vi "Commercial2 Dryer Tool.vi"() -> ()   [LabVIEW 2023]
uses:
  Common/LabVIEW GEA2 Toolkit/GEA3/type defs/Data In.ctl
  Common/LabVIEW GEA2 Toolkit/GEA3/type defs/Source_Destination.ctl
  Common/LabVIEW GEA2 Toolkit/GEA3/type defs/ERD Write Data In.ctl
  Common/LabVIEW GEA2 Toolkit/GEA3/type defs/Data Type.ctl
  Common/LabVIEW GEA2 Toolkit/GEA3/type defs/ERD Read Data Out.ctl
  Common/LabVIEW GEA2 Toolkit/GEA3/type defs/ERD Read Data In.ctl
  Common/type defs/Programming.ctl
  Common/type defs/Flash_Results.ctl
  JL Dryer Tool Support/type defs/Cycle Control.ctl
  JL Dryer Tool Support/type defs/ERD_Always_Show_JL.ctl
  Common/GEA2 Script/typedefs/Script Info.ctl
  JL Dryer Tool Support/type defs/Relay_Control.ctl
  JL Dryer Tool Support/type defs/Drum_Light_Control.ctl
  <vilib>/Platform/fileVersionInfo.llb/FileVersionInformation.ctl
  Common/type defs/Choose_ERD_List.ctl
  Common/Diagnostics Decode/Type Defs/Diag_FaultTableStatus.ctl
  Common/Diagnostics Decode/Type Defs/Diag_FaultTableEntry.ctl
  Common/Diagnostics Decode/Type Defs/Diag_EntityManifestType.ctl
  Common/Diagnostics Decode/Type Defs/Diag_FaultSeqEntry.ctl
  Automation2/Product Specific/Clothes Care/Justice League/Product Testcode/Diagnostics/TypeDefs/Centauro Diagnostic V3 SnapShot.ctl
  JL Dryer Tool Support/type defs/JL_Diagnost V3 Cycle History.ctl
  Common/type defs/ERDList.ctl
  Common/type defs/ERD_Loop_States.ctl
  JL Dryer Tool Support/type defs/ERD_Commercial_Laundry.ctl
  JL Dryer Tool Support/type defs/ERD_RJ45.ctl
  Common/type defs/Version.ctl
  Common/type defs/BootloaderVersion.ctl
  Common/LabVIEW GEA2 Toolkit/GEA3/type defs/Data Out.ctl
  Common/type defs/ERD_Data_Loop_Control.ctl
  Common/type defs/Error_Command.ctl
  JL Dryer Tool Support/type defs/All_Bundled_Data_JL.ctl
  Common/type defs/CSV_File_String_Arrays.ctl
  Common/type defs/Fault Table Array.ctl
  Common/type defs/Fault_Table_Info.ctl
  JL Dryer Tool Support/type defs/Heat Control.ctl
  Common/GExplorer Support/typedefs/GExplorer_Data_Cluster.ctl
  JL Dryer Tool Support/type defs/DAQ_Control_Command.ctl
  Common/type defs/ERD_Loop_Control_Command.ctl
  Common/type defs/GEA2_Control_Command.ctl
  Common/LabVIEW GEA2 Toolkit/GEA3/advanced/GEA2 Message Received Event Handler.vi
  D:/Common/LabVIEW GEA2 Toolkit/source/GEA3 DLL Source/GeaCommunication.dll
  Common/LabVIEW GEA2 Toolkit/source/GEA3 DLL Source/GeaCommunication.dll
  Common/LabVIEW GEA2 Toolkit/GEA3/library/GEA2_Toolkit.lvlib
panel:
  out "Message":string
  in  "EndOfCycle":bool
  in  "Board Index":u8=1 max=10 step=1
  in  "Pause(mls)":u32=100
  out "Rate":u32=100
  out "State":T1=enum."Read ERDs"
  out "ERD_Always Show":T2={"Inlet Thermistor"=0, "Machine State"="IDLE", "Filtered Moisture"=0, "Cycle Selected"="", "HTR 1 / Inner / Top"=FALSE, "HTR 2 / Outer / Bot"=FALSE, "Door Switch"=FALSE, "Drum Light"=FALSE, "Cycle Engine State"="", "Centrifugal Switch"=FALSE, "Drum Motor"=FALSE, "Cycle Count"=0, "Ext. Tumble"=FALSE, "eDry"=FALSE, "Temp Level"="", "Dryness Level"="", "Time Level"="", "Delay Time (min)"=0, "Steam Refresh"=FALSE, "Damp Alert"=FALSE, "Sub-Cycle"="", "Outlet Thermistor"=0, "Target Moisture"=0, "Remaining Cycle Time"=0, "Raw Moisture"=0, "Cycle Name"="", "My Cycle"=FALSE, "Delay Dry"=FALSE, "Detangle"=FALSE, "Control Lock"=FALSE, "Steam Valve"=FALSE, "Door Latch"=FALSE, "Signal Volume"="", "Tune ID"="", "Restr Detect Status"="", "Vent Restriction"="", "Load Size by Contact"="", "Load Size by Temp"="", "EOC Reason"="", "Sensor Dry Status"="", "Dampness State"="", "Target Voltage Reached"=FALSE, "TrimInhibitR1"=FALSE, "TrimInhibitR2"=FALSE, "TrimBothCoilInhibit"=FALSE, "NormalHeatControl"=FALSE, "HeatControl Request"=FALSE, "Cool Down Status"="", "EcoDryInhibitRelay1"=FALSE, "EcoDryInhibitRelay2"=FALSE, "ReverseDrumInhibitRelay1"=FALSE, "ReverseDrumInhibitRelay2"=FALSE, "OverTempHeaterInhibitRequest"=FALSE, "FallbackHeatControlMethodStatus"=FALSE, "IHC TimeSeconds"=0, "ECT TimeSeconds "=0, "SC Total Drying Time(S')"=0, "TTR Target Voltage (S')"=0, "TCT Drying Time (S's)"=0, "Drum Motor State"=enum."Off", "Load Size by Ag"="", "MaxFIletered Voltage"=0, "Dry Load Detection"="", "Min Sensing Elapse Sec"=0, "Time Multi Sec X100"=0, "Time Adder  Sec"=0, "Temp Multi EcoDry"="", "Temp Multi ExtraLow"="", "Temp Multi Low "="", "Temp Multi Medium"="", "Temp Multi High"="", "SmoothMoisture"=0, "Eco Dry SEL Status"="", "Eco Dry SEL Result"="", "Eco Dry Cont Status"="", "Eco Dry Relay1 Timer"="", "Eco Dry Relay2 Timer "="", "Eco Dry Stage 2 Tans "=0, "WiFiCommissioningPSt"="IDLE", "Payment Method"=""}
  out "Temp ADC":T3
  in  "Read Parametric":bool=TRUE
  in  "Data ON":bool=TRUE
  in  "Stop":bool
  in  "Reset":bool
  in  "UI Launch":bool
  in  "Tab Control":T4(tab)=enum."ERD List"
  in  "Phase.Authorized":bool
  in  "Phase.Reserved":bool
  in  "Phase.Idle":bool
  in  "Residencial":bool
  out "Personality Set":u8=1
  in  "?":u8=1
  in  "Set Personality":bool
  out "CSV File Log Path":path=path "D:/QA/Commercial 2/Dryer_Xolo/ProbandoC2_24-11-21_15-05-37.csv"
  out "Commercial_Laundry":T5
  out "RJ45":T6
  out "Version":T7
  in  "Read ERD List":T8[](array[typedef])=[{"ERD Number"=49, "Data Type"=enum."string"}] {"ERD Number" format="%.0x"}
  in  "Read ERD":bool
  in  "Write ERD List":T9[](array[typedef])=[{"ERD Number"=49, "Data Type"=enum."string", "Data"="01"}] {"ERD Number" format="%.0x"}
  in  "Write ERD":bool
  out "Read ERD Data Out":T11[](array[typedef])=[{"ERD Number"=49, "Data"="00 00 00 16"}] {"ERD Number" format="%.0x"}
  out "Boot Loader Version":T12
  in  "GEA Inputs":T13={"Source"=229, "Destination"=192} {"Destination" format="%.0x"; "Source" format="%.0x"}
  out "Increment Price":T14={"DELICATE"=0.0, "LOW"=0.0, "MEDIUM"=0.5, "HIGH"=0.25} {"HIGH" min=0.0 max=9.75 step=0.25; "MEDIUM" min=0.0 max=9.75 step=0.25; "LOW" min=0.0 max=9.75 step=0.25; "DELICATE" min=0.0 max=9.75 step=0.25}
  out "Base Price":T14={"DELICATE"=0.0, "LOW"=0.0, "MEDIUM"=0.5, "HIGH"=0.25} {"HIGH" min=0.0 max=9.75 step=0.25; "MEDIUM" min=0.0 max=9.75 step=0.25; "LOW" min=0.0 max=9.75 step=0.25; "DELICATE" min=0.0 max=9.75 step=0.25}
  in  "See Price":bool
  in  "IncrementPrices":T14={"DELICATE"=0.0, "LOW"=0.25, "MEDIUM"=0.5, "HIGH"=0.25} {"HIGH" min=0.0 max=9.75 step=0.25; "MEDIUM" min=0.0 max=9.75 step=0.25; "LOW" min=0.0 max=9.75 step=0.25; "DELICATE" min=0.0 max=9.75 step=0.25}
  in  "SetIncrementPrices":bool
  in  "BasePrices":T14={"DELICATE"=0.0, "LOW"=0.0, "MEDIUM"=0.5, "HIGH"=0.25} {"HIGH" min=0.0 max=9.75 step=0.25; "MEDIUM" min=0.0 max=9.75 step=0.25; "LOW" min=0.0 max=9.75 step=0.25; "DELICATE" min=0.0 max=9.75 step=0.25}
  in  "Set Price":bool
  out "Increment Time":T15 {"HIGH" max=10 step=1; "MEDIUM" max=10 step=1; "LOW" max=10 step=1; "DELICATE" max=10 step=1}
  out "Base Time":T15 {"HIGH" max=10 step=1; "MEDIUM" max=10 step=1; "LOW" max=10 step=1; "DELICATE" max=10 step=1}
  in  "See Times":bool
  in  "Time Increment":T14={"DELICATE"=0.0, "LOW"=0.0, "MEDIUM"=1.0, "HIGH"=0.0} {"HIGH" min=0.0 max=90.0 step=1.0; "MEDIUM" min=0.0 max=90.0 step=1.0; "LOW" min=0.0 max=90.0 step=1.0; "DELICATE" min=0.0 max=90.0 step=1.0}
  in  "SetTimeIncrement":bool
  in  "Time Base":T16={"DELICATE"=0.0, "LOW"=10.0, "MEDIUM"=10, "HIGH"=10} {"HIGH" min=10 max=90 step=1; "MEDIUM" min=10 max=90 step=1; "LOW" min=10.0 max=90.0 step=1.0; "DELICATE" min=0.0 max=90.0 step=1.0}
  in  "Set Base Time":bool
  out "OK?":bool
  in  "Parametric":T17(ring)
  in  "Exit Botloader":bool
  in  "Enum":enum16{"All", "MC", "UI"}(ring)
  in  "Entry Botloader":bool
  out "FileVersionInfo":T18
  out "LabView/Version Number":string
  in  "Tool Version":bool=TRUE
  in  "Clear":bool
  in  "Programming":T19={"Program"=FALSE, "File Path"=path "", "Program Ind"=FALSE, "Reset Board"=FALSE, "Enter Bootloader"=FALSE, "Result"=9} {"Result" items=["ImageRejected", "BoardNotFound", "UnableToGetGeaConfiguration", "WriteToFlashNotAllowed", "ImageDownloadedSuccessfully", "ImagePresent", "WriteToFlashFailed", "EraseFailed", "CrcFailed", ""]}
  in  "Flash Latest":bool
  in  "Send Button":bool
  in  "GEA2 Send":T21={"Source"=228, "Destination"=192, "Command"=0, "Message"=""} {"Command" format="%02x"; "Destination" format="%02x"; "Source" format="%02x"}
  out "Converted Data Out":T22 {"CRC" format="%04x"; "Length" format="%02x"; "Command" format="%02x"; "Destination" format="%02x"; "Source" format="%02x"}
  in  "Write parametric":bool
  in  "Message to send":string="04 03"
  in  "Get Faults":bool
  in  "Clear Fault Table Buffer":bool
  in  "Clear Fault Seq Buffer":bool
  out "Fault Sequence Entries":T23[](array[typedef])
  out "Fault Seq Status":T24
  out "Fault Table Entries":T25[](array[typedef])
  out "Fault Table Status":T24
  out "Diagnostic Entity Manifest":T26
  out "Major Version":u8
  out "Minor Version":u8
  out "Fault Set?":bool
  in  "Filter by Count":bool=TRUE
  out "Centauro Fault Snapshot":T27
  in  "Drum Light":T28={"Drum Light ON"=FALSE, "Drum Light OFF"=FALSE, "On Time (s)"=5.0} {"On Time (s)" min=0.0 max=3600.0}
  in  "Relay Control":T29
  in  "LED Control":T30
  in  "Cycle Control":T31
  out "Sensor Dry Status":string
  out "Dampness State":string
  in  "Enable CC Mode":bool
  in  "Completed Cycles":u16
  in  "Requested Cycles":u16
  in  "TimeBetween Cycles":u32
  in  "Enabled":u8
  in  "ERD Spam GEA Inputs":T13={"Source"=229, "Destination"=192} {"Destination" format="%.0x"; "Source" format="%.0x"}
  in  "Get Cycle Data":bool
  in  "Filter by Status Count":bool=TRUE
  out "JL Cycle History":T32
  out "output cluster":T24
  in  "Script Log Path":path
  in  "Run Script":bool
  out "Script Pass/Fail?":bool
  out "Script Report Text":string
  in  "stop script":bool
  in  "Script Path":path
  out "Script Info":T33 {"Overall Script File Progress" scale=0.0..1.0; "Elapsed time (s)" format="%#.1f"; "Current Script Progress" scale=0.0..1.0}
  out "Script Error Out":errorcluster
  in  "Load ERD List":T34
  in  "ERD Default List":T35=[{"Boolean"=TRUE, "ERD Number"=8192, "ERD Nanme"="Erd_MachineStatus", "Data_Type"=enum."string"}, {"Boolean"=TRUE, "ERD Number"=65281, "ERD Nanme"="Erd_Personality", "Data_Type"=enum."string"}, {"Boolean"=TRUE, "ERD Number"=65423, "ERD Nanme"="Erd_EnterConsumerErrorMode", "Data_Type"=enum."string"}, {"Boolean"=TRUE, "ERD Number"=55, "ERD Nanme"="Erd_ServiceModeState", "Data_Type"=enum."string"}, {"Boolean"=TRUE, "ERD Number"=61811, "ERD Nanme"="EErd_WiFiCommissioningOption", "Data_Type"=enum."string"}, {"Boolean"=TRUE, "ERD Number"=61823, "ERD Nanme"="Erd_WiFiCommissioningPresenterState", "Data_Type"=enum."string"}, {"Boolean"=TRUE, "ERD Number"=55, "ERD Nanme"="Erd_ServiceModeState", "Data_Type"=enum."string"}, {"Boolean"=TRUE, "ERD Number"=61811, "ERD Nanme"="Erd_WiFiCommissioningOption", "Data_Type"=enum."string"}, {"Boolean"=TRUE, "ERD Number"=65522, "ERD Nanme"="Erd_Rj45LockedAtLeastOnce", "Data_Type"=enum."string"}, {"Boolean"=TRUE, "ERD Number"=8351, "ERD Nanme"="Erd_CommercialLaundryStatus", "Data_Type"=enum."string"}, {"Boolean"=TRUE, "ERD Number"=8350, "ERD Nanme"="Erd_CommercialLaundryStatusExternal", "Data_Type"=enum."string"}, {"Boolean"=TRUE, "ERD Number"=8398, "ERD Nanme"="Erd_RJ45WriteAccessActual", "Data_Type"=enum."string"}, {"Boolean"=TRUE, "ERD Number"=8397, "ERD Nanme"="Erd_RJ45WriteAccessRequest", "Data_Type"=enum."string"}, {"Boolean"=TRUE, "ERD Number"=61976, "ERD Nanme"="Erd_CommercialPaymentMethod", "Data_Type"=enum."string"}, {"Boolean"=TRUE, "ERD Number"=61977, "ERD Nanme"="Erd_CommercialCoinPaymentStatusRequest", "Data_Type"=enum."string"}] {"ERD Number" format="%x"}
  in  "ERD's List Ticket Testing":T35 {"ERD Number" format="%x"}
  in  "Wifi State":T36(ring)
  in  "Set Wifi State(ERD 6003)":bool
  in  "Turn on Wifi":bool
  in  "Turn off Wifi":bool
  out "Wifi Network State":string
  out "Wifi Password":string
  out "Wifi Network Name":string
  out "Mac Address":string
  in  "Get Wifi Data":bool
  out "Error Out":errorcluster
  # "Personality"
  # "Residencial"
  # "Simular pago con aplicación 209E phase"
  # "Ver. 1.3"
  # "Set Base Prices"
  # "BASE"
  # "INCREMENT"
  # "Set Increment Prices"
  # "Set Time Base"
  # "BASE"
  # "INCREMENT"
  # "Set Time Increments"
  # "This controls destination of ERD Spam.\nYou should never change source unless\nyou want to see the spam in the GEA log."
  # "Continuous cycle Config"
  # "Wifi State is Writing to ERD 6003 and communicating with the wifi board directly.  It will remain in the state you wrote it to until another command is recieved. \n\nOnly Write to invalid if you are testing the board in Invalid state."
  # "After turning on Wifi , wait about 30 seconds and press the Get Wifi Data button.  Network state should be 1, apmode.\n\nAll this is doing is Writing the ERD 0xF115 Service Request to request connect, or disconnect."
  # "Contact:\n\nTerrance Bradford\nTerrance.Bradford@geappliances.com"
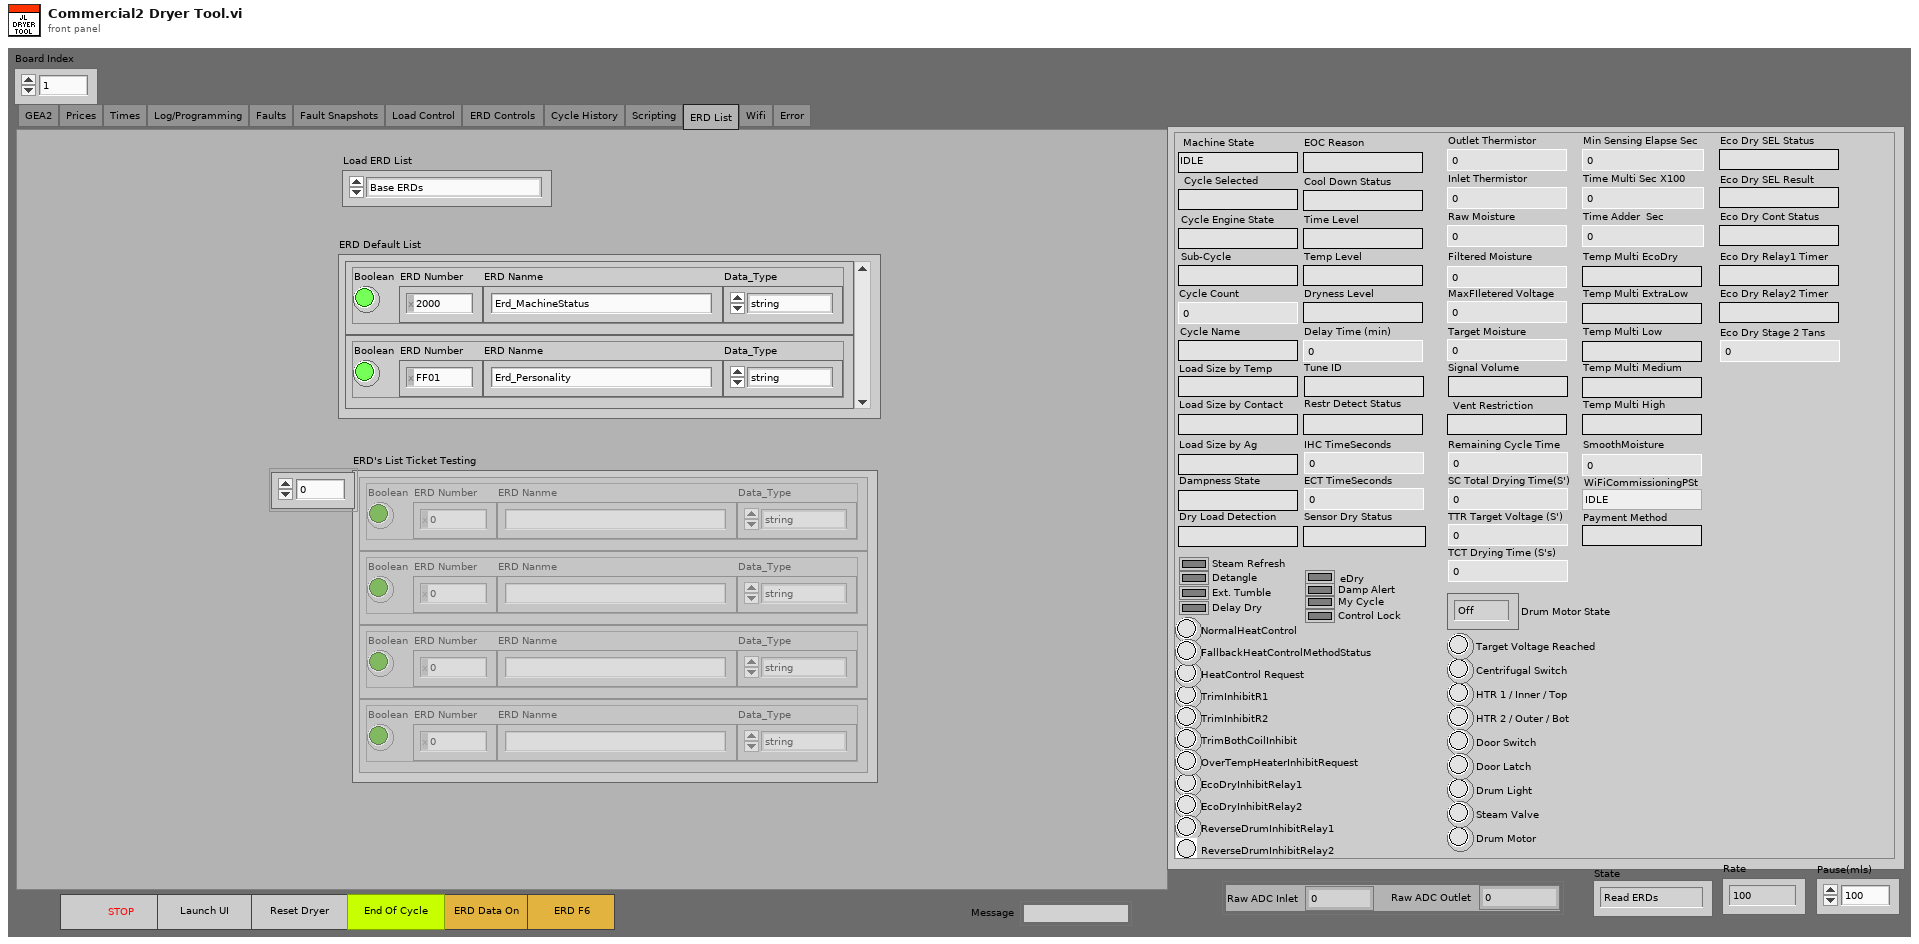
[diagram p1: front panel]
types:
  T1 = typedef "ERD_Loop_States.ctl" = enum16{"Init", "Build ERD Read List", "Read ERDs", "Get Version", "ERD´s User show", "Update UI", "Graph", "Read Faults", "Log Data", "Pause", "Shutdown"}
  T2 = typedef "ERD_Always_Show_JL.ctl" = cluster{"Inlet Thermistor":u16, "Machine State":string, "Filtered Moisture":u16, "Cycle Selected":string, "HTR 1 / Inner / Top":bool, "HTR 2 / Outer / Bot":bool, "Door Switch":bool, "Drum Light":bool, "Cycle Engine State":string, "Centrifugal Switch":bool, "Drum Motor":bool, "Cycle Count":u32, "Ext. Tumble":bool, "eDry":bool, "Temp Level":string, "Dryness Level":string, "Time Level":string, "Delay Time (min)":u16, "Steam Refresh":bool, "Damp Alert":bool, "Sub-Cycle":string, "Outlet Thermistor":u16, "Target Moisture":u16, "Remaining Cycle Time":u32, "Raw Moisture":u16, "Cycle Name":string, "My Cycle":bool, "Delay Dry":bool, "Detangle":bool, "Control Lock":bool, "Steam Valve":bool, "Door Latch":bool, "Signal Volume":string, "Tune ID":string, "Restr Detect Status":string, "Vent Restriction":string, "Load Size by Contact":string, "Load Size by Temp":string, "EOC Reason":string, "Sensor Dry Status":string, "Dampness State":string, "Target Voltage Reached":bool, "TrimInhibitR1":bool, "TrimInhibitR2":bool, "TrimBothCoilInhibit":bool, "NormalHeatControl":bool, "HeatControl Request":bool, "Cool Down Status":string, "EcoDryInhibitRelay1":bool, "EcoDryInhibitRelay2":bool, "ReverseDrumInhibitRelay1":bool, "ReverseDrumInhibitRelay2":bool, "OverTempHeaterInhibitRequest":bool, "FallbackHeatControlMethodStatus":bool, "IHC TimeSeconds":u32, "ECT TimeSeconds ":u32, "SC Total Drying Time(S')":u32, "TTR Target Voltage (S')":u32, "TCT Drying Time (S's)":u32, "Drum Motor State":enum16{"Off", "Cw", "Ccw", "Max"}, "Load Size by Ag":string, "MaxFIletered Voltage":u16, "Dry Load Detection":string, "Min Sensing Elapse Sec":u32, "Time Multi Sec X100":u32, "Time Adder  Sec":u32, "Temp Multi EcoDry":string, "Temp Multi ExtraLow":string, "Temp Multi Low ":string, "Temp Multi Medium":string, "Temp Multi High":string, "SmoothMoisture":u16, "Eco Dry SEL Status":string, "Eco Dry SEL Result":string, "Eco Dry Cont Status":string, "Eco Dry Relay1 Timer":string, "Eco Dry Relay2 Timer ":string, "Eco Dry Stage 2 Tans ":u32, "WiFiCommissioningPSt":string, "Payment Method":string}
  T3 = cluster{"Raw ADC Outlet":u16, "Raw ADC Inlet":u16}
  T4 = enum32{"GEA2", "Prices", "Times", "Log/Programming", "Faults", "Fault Snapshots", "Load Control", "ERD Controls ", "Cycle History", "Scripting", "ERD List", "Wifi", "Error"}
  T5 = typedef "ERD_Commercial_Laundry.ctl" = cluster{"Session":string, "Phase":string, "Appliance Type":string, "Cycle Selected":string, "Platform Type":string, "Retry Signal":string, "Session Ext":string, "Phase Ext":string, "Appliance Type Ext":string, "Cycle Selected Ext":string, "Platform Type Ext":string, "Retry Signal Ext":string}
  T6 = typedef "ERD_RJ45.ctl" = cluster{"Write Access Actual":string, "Write Access Request":string, "LockedAtLeastOnce":string}
  T7 = typedef "Version.ctl" = cluster{"Build Number":string, "Build Hash ":string, "Application Version":string, "Parametric Version":string, "UI App Version":string}
  T8 = typedef "ERD Read Data In.ctl" = cluster{"ERD Number":u16, "Data Type":enum16{"string", "boolean", "uint8_t", "uint16_t", "uint32_t", "uint64_t", "int8_t", "int16_t", "int32_t", "int64_t"}}
  T9 = typedef "ERD Write Data In.ctl" = cluster{"ERD Number":u16, "Data Type":T10, "Data":string}
  T10 = typedef "Data Type.ctl" = enum16{"string", "boolean", "uint8_t", "uint16_t", "uint32_t", "uint64_t", "int8_t", "int16_t", "int32_t", "int64_t"}
  T11 = typedef "ERD Read Data Out.ctl" = cluster{"ERD Number":u16, "Data":string}
  T12 = typedef "BootloaderVersion.ctl" = cluster{"UI BL Version":string, "MC BL Version":string}
  T13 = typedef "Source_Destination.ctl" = cluster{"Source":u8, "Destination":u8}
  T14 = cluster{"DELICATE":dbl, "LOW":dbl, "MEDIUM":dbl, "HIGH":dbl}
  T15 = cluster{"DELICATE":u32, "LOW":u32, "MEDIUM":u32, "HIGH":u32}
  T16 = cluster{"DELICATE":dbl, "LOW":dbl, "MEDIUM":u8, "HIGH":u8}
  T17 = enum16{"Board SKU", "Board Serial Number", "Unit SKU", "Unit Serial Number"}
  T18 = typedef "FileVersionInformation.ctl" = cluster{"FileVersion":string, "ProductName":string, "InternalName":string, "CompanyName":string, "LegalCopyright":string, "FileDescription":string}
  T19 = typedef "Programming.ctl" = cluster{"Program":bool, "File Path":path, "Program Ind":bool, "Reset Board":bool, "Enter Bootloader":bool, "Result":T20}
  T20 = typedef "Flash_Results.ctl" = i32
  T21 = typedef "Data In.ctl" = cluster{"Source":u8, "Destination":u8, "Command":u8, "Message":string}
  T22 = typedef "GEA2_Toolkit.lvlib/Data Out.ctl" = cluster{"Source":u8, "Destination":u8, "Command":u8, "Length":u8, "CRC":u16, "Message":string}
  T23 = typedef "Diag_FaultSeqEntry.ctl" = cluster{"Cycle #":u32, "Time":u32, "F Code":string, "F Active":bool}
  T24 = typedef "Diag_FaultTableStatus.ctl" = cluster{"Cur Index":u16, "Count":u16, "Ov Cnt":u16}
  T25 = typedef "Diag_FaultTableEntry.ctl" = cluster{"Cycle #":u32, "Time":u32, "F Code":string, "F Count":u16, "F Active":bool}
  T26 = typedef "Diag_EntityManifestType.ctl" = cluster{"ID":u8, "Data Ver Maj":u8, "Data Ver Min":u8, "Fault Table?":bool, "Fault Table Snap?":bool, "Fault Seq?":bool, "Fault Seq Snap?":bool, "Cycle History Seq?":bool, "Fault Table Entry Count":u16, "Fault Seq Entry Count":u16, "Cycle History Entry Count":u16, "Cycle Count":u32, "Entity Run Time (Min)":u32}
  T27 = typedef "Centauro Diagnostic V3 SnapShot.ctl" = string[][]
  T28 = typedef "Drum_Light_Control.ctl" = cluster{"Drum Light ON":bool, "Drum Light OFF":bool, "On Time (s)":dbl}
  T29 = typedef "Relay_Control.ctl" = cluster{"Drum Motor":bool, "HTR 2 / Outer / Bot":bool, "Steam Valve":bool, "Relays ON":bool, "Relays OFF":bool, "HTR 1 / Inner / Top":bool, "Pump":bool}
  T30 = cluster{"ALL LEDs ON":bool, "ALL LEDs OFF":bool, "Reset LEDs":bool}
  T31 = typedef "Cycle Control.ctl" = cluster{"Start Cycle":bool, "Cycle Selection":u8, "Stop Cycle":bool, "Pause Cycle":bool, "Resume Cycle":bool, "Select Cycle":bool}
  T32 = typedef "JL_Diagnost V3 Cycle History.ctl" = string[][]
  T33 = typedef "Script Info.ctl" = cluster{"Overall Script File Progress":dbl, "Current Script Progress":dbl, "Script":string, "Test":string, "Elapsed time (s)":dbl, "Done?":bool}
  T34 = typedef "Choose_ERD_List.ctl" = enum16{"Base ERDs", "QA ERDs", "MABE ERD List", "EcoDry Evaluation ERD List", "ClothDampnessCheck ERD List"}
  T35 = typedef "ERDList.ctl" = cluster{"Boolean":bool, "ERD Number":u16, "ERD Nanme":string, "Data_Type":enum16{"string", "boolean", "uint8_t", "uint16_t", "uint32_t", "uint64_t", "int8_t", "int16_t", "int32_t", "int64_t"}}[]
  T36 = enum16{"0 - OFF", "1 - App Mode", "2 - Connecting", "3 - Connected", "4 - Connected Off", "5 - Scanning", "6 - Reconnecting", "255 - Invalid"}
  T37 = typedef "All_Bundled_Data_JL.ctl" = cluster{"Version":T7, "ERD_Always Show":T2, "Personality Set":u8, "CSV File String Arrays":T38, "Fault Table Array ":T39, "Heat Control":T41, "Temp ADC":cluster{"Raw ADC Outlet":u16, "Raw ADC Inlet":u16}, "Commercial_Laundry":T5, "Boot Loader Version":T12, "RJ45":T6}
  T38 = typedef "CSV_File_String_Arrays.ctl" = cluster{"ERD Number Array":string[], "ERD Name Array":string[], "ERD Converted String Data":string[]}
  T39 = typedef "Fault Table Array.ctl" = T40[]
  T40 = typedef "Fault_Table_Info.ctl" = cluster{"Cycle Count":u32, " Runtime (min) ":u32, "Fault Status":string, "Fault ID":string, "Fault Count":u16}
  T41 = typedef "Heat Control.ctl" = cluster{"Htr1 InletLowLim":string, "Htr1 InletUpLim":string, "Htr1 OutletLowLim":string, "Htr1 OutletUpLim":string, "Htr1 FallBackON(s)":string, "Htr1 FallBackOFF(s)":string, "Htr1":bool, "Htr2 InletLowLim":string, "Htr2 InletUpLim":string, "Htr2 OutletLowLim":string, "Htr2 OutletUpLim":string, "Htr2 FallBackON(s)":string, "Htr2 FallBackOFF(s)":string, "Htr2":bool}
  T42 = typedef "ERD_Data_Loop_Control.ctl" = cluster{"Data":variant, "State":T1}
  T43 = typedef "Error_Command.ctl" = enum16{"Initialize", "Handle Errors", "Report Errors"}
  T44 = enum8{"Enabled", "Disabled", "Disabled and Grayed Out"}
  T45 = enum16{"UI Application APL", "UI Parametric APL", "MC APL"}
  T46 = typedef "GEA2_Control_Command.ctl" = enum16{"Initialize", "Shutdown"}
  T47 = typedef "ERD_Loop_Control_Command.ctl" = enum16{"Initialize", "Shutdown"}
  T48 = typedef "DAQ_Control_Command.ctl" = enum16{"Initialize", "Shutdown", "Exit"}
  T49 = typedef "GExplorer_Data_Cluster.ctl" = cluster{"Data":variant, "State":enum16{"Add to Log", "Clear", "Shutdown"}}
  T50 = typedef "F6_ERD_Control.ctl" = cluster{"EcoDryEnabledFlag":string, "KeyCycleId":u8, "CycleType":string, "Time LVL option 5":u32, "Time LVL option 4":u32, "Time LVL option _3":u32, "Time LVL option _2":u32, "Time LVL option _1":u32, "Time LVL option _0":u32, "CoolDownTimeInSeconds":u32, "TimeAdjustTimeCycleMinimumTimeInSeconds":u32, "TimeAdjustTimeCycleMaximumTimeInSeconds":u32, "TimeAdjustTimeCycleStandardAdjustTimeInSeconds":u32, "TimeAdjustTimeCycleSlewAdjustTimeInSeconds":u32, "ExtendedTumbleTimeInSeconds":u32, "SanitizeMaxDryTimeInSeconds":u32, "TemperatureDefault Level":u8, "Temperature ecoDryDefualtLevel":u8, "DrynessDefault Level":u8, "DrynessDefault ecoDryDefualtLevel":u8, "TimeAdjust defaultLevel":u8, "TimeAdjust ecoDryDefualtLevel":u8, "TimeLevelDefault Level":u8, "TimeLevelDefault Eco Dry":u8, "EStarSensorDry Default Level":u8, "EStarSensorDry ecoDryDefaultLevel":u8, "EcoDryDefault Level":u8, "EcoDryDefault EcoDryDefaultLevel ":u8, "ExtendedTumble Default Level":u8, "ExtendedTumble  EcoDryDefaultLevel":u8, "Sanitize Default Level":u8, "Sanitize ecoDryDefualtLevel":u8, "MyCycleDefault Level":u8, "MyCycleDefault ecoDryDefualtLevel":u8, "StartPause Default Level":u8, "StartPause ecoDryDefualtLevel":u8, "Power Default Level":u8, "Power ecoDryDefualtLevel":u8, "KeyVolume Default Level":u8, "KeyVolume ecoDryDefualtLevel":u8, "AlertVolume Default Level":u8, "AlertVolume ecoDryDefualtLevel":u8, "ControlLock Default Level":u8, "ControlLock EecoDryDefualtLevel":u8, "HeatControlRelay1EcoDryParametricDataEntry\nHeatControlTemperatureLimit_InletLower":u16, "HeatControlRelay1EcoDryParametricDataEntry\nHeatControlTemperatureLimit_InletUpper":u16, "HeatControlRelay1EcoDryParametricDataEntry\nHeatControlTemperatureLimit_OutletLower":u16, "HeatControlRelay1EcoDryParametricDataEntry\nHeatControlTemperatureLimit_OutletUpper":u16, "HeatControlRelay1EcoDryParametricDataEntry\nonTimeInSeconds":u8, "HeatControlRelay1EcoDryParametricDataEntry\noffTimeInSeconds":u8, "HeatControlRelay1EcoDryParametric\nDataEntryChange ":bool, "HeatControlRelay2 EcoDryParametricDataEntry\nHeatControlTemperatureLimit_InletLower":u16, "HeatControlRelay2 EcoDryParametricDataEntry\nHeatControlTemperatureLimit_InletUpper ":u16, "HeatControlRelay2EcoDryParametricDataEntry\nHeatControlTemperatureLimit_OutletLower ":u16, "HeatControlRelay2EcoDryParametricDataEntry\nHeatControlTemperatureLimit_OutletUpper":u16, "HeatControlRelay2EcoDryParametricDataEntry\nonTimeInSeconds ":u8, "HeatControlRelay2EcoDryParametricDataEntry\noffTimeInSeconds ":u8, "HeatControlRelay2EcoDry\nParametricDataEntryChange":bool, "DampAlert Default Level":u8, "DampAlert ecoDryDefaultLevel":u8, "Detangle Default Level ":u8, "Detangle ecoDryDefaultLevel":u8, "DelayStart Default Level":u8, "DelayStart ecoDryDefaultLevel":u8, "CycleAllowsInventoryChangeChange":bool, "TemperatureAllowable":u8, "DrynessAllowable":u8, "TimeLevelAllowable":u8, "EcoDryAllowable":u8, "ExtendedTumbleAllowable":u8, "DampAlertAllowable":u8, "DetangleAllowable":u8, "DelayStartAllowable":u8, "SanitizeAllowable":u8, "MyCycleAllowable":u8, "TimeAdjustAllowable":u8, "Power Allowable":u8, "KeyVolumeAllowable":u8, "AlertVolumeAllowable":u8, "ControlLockAllowable":u8, "EStarSensorDryAllowable":string, "StartPauseAllowable":u8, "EcoDryStage1Heater2\nActiveSeconds":u32, "EcoDryStage2PeriodSeconds":u32, "EcoDryStage2Heater1\nActiveSeconds":u32, "EcoDryStage2Heater2\nActiveSeconds":u32, "EcoDryStage1Heater1\nActiveSeconds":u32, "EcoDryStage1PeriodSeconds":u32, "EcoDryStage2DurationSeconds":u32, "CoolDownAdaptiveTargetTemperature":u16}
  T51 = enum32{"invalid app kind", "Development System", "Run Time System", "Student Edition", "Embedded LabVIEW", "Evaluation", "Custom"}
  T52 = cluster{"ERD Data Out[0]":cluster{"ERD Number":u16, "Data":string}, "ERD Data Out[1]":cluster{"ERD Number":u16, "Data":string}, "ERD Data Out[2]":cluster{"ERD Number":u16, "Data":string}, "ERD Data Out[3]":cluster{"ERD Number":u16, "Data":string}, "ERD Data Out[4]":cluster{"ERD Number":u16, "Data":string}, "ERD Data Out[5]":cluster{"ERD Number":u16, "Data":string}, "ERD Data Out[6]":cluster{"ERD Number":u16, "Data":string}, "ERD Data Out[7]":cluster{"ERD Number":u16, "Data":string}, "ERD Data Out[8]":cluster{"ERD Number":u16, "Data":string}}
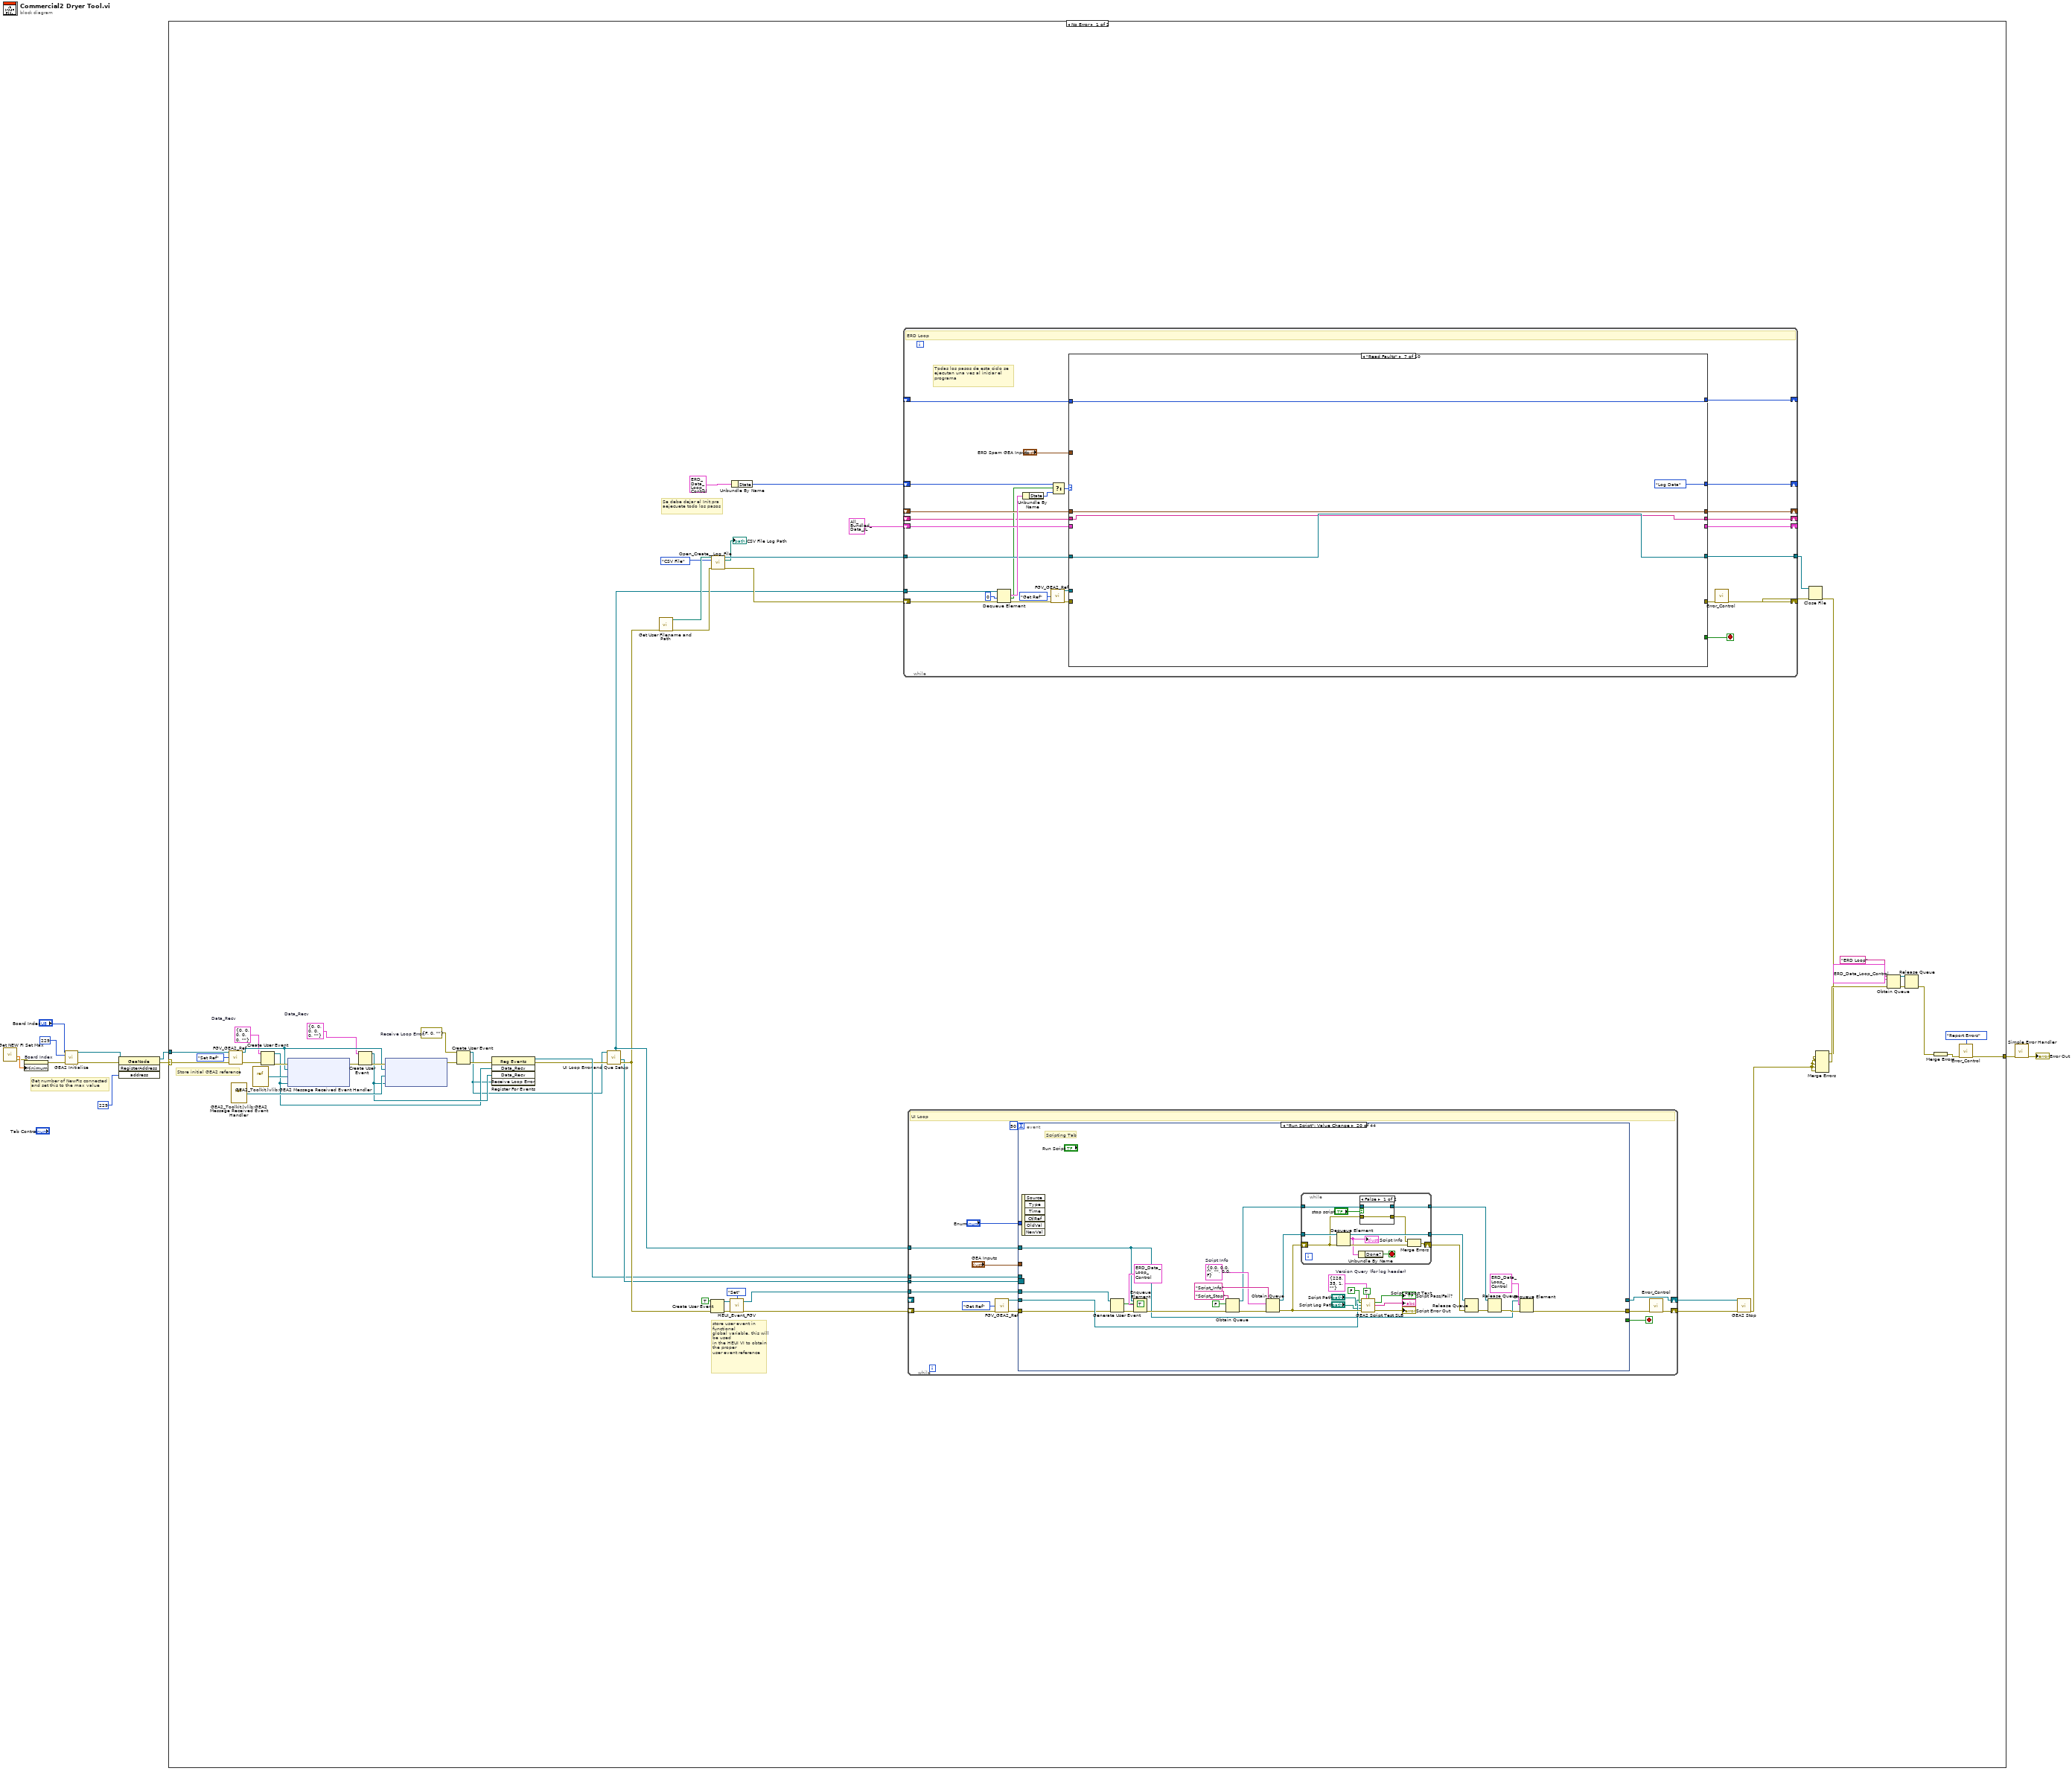
[diagram p0: block diagram]
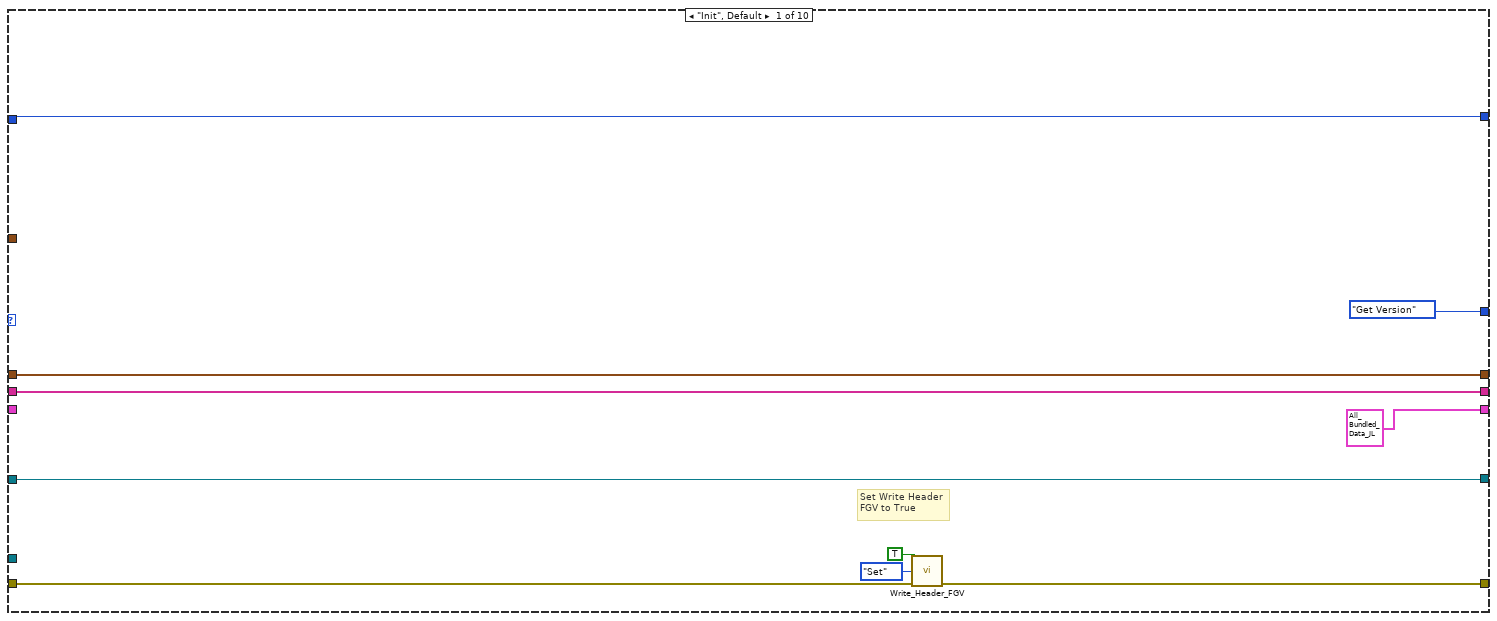
[diagram p2: hidden frame]
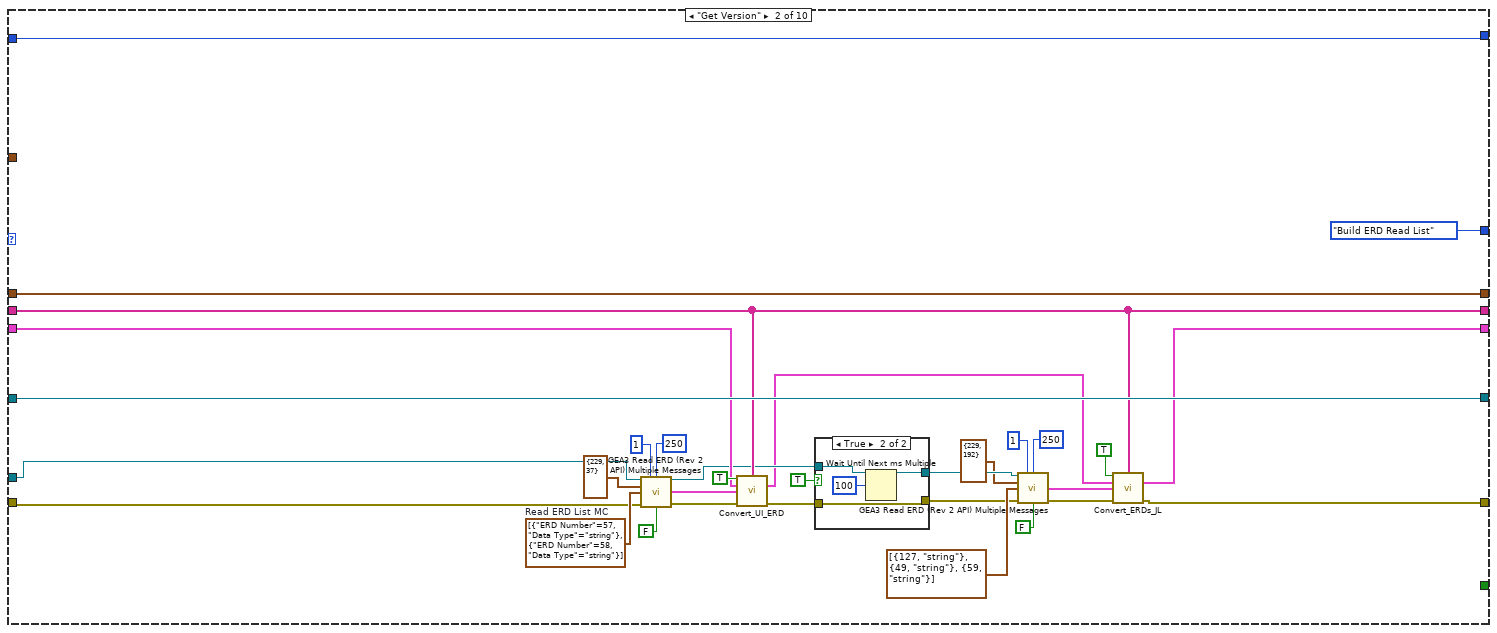
[diagram p3: hidden frame]
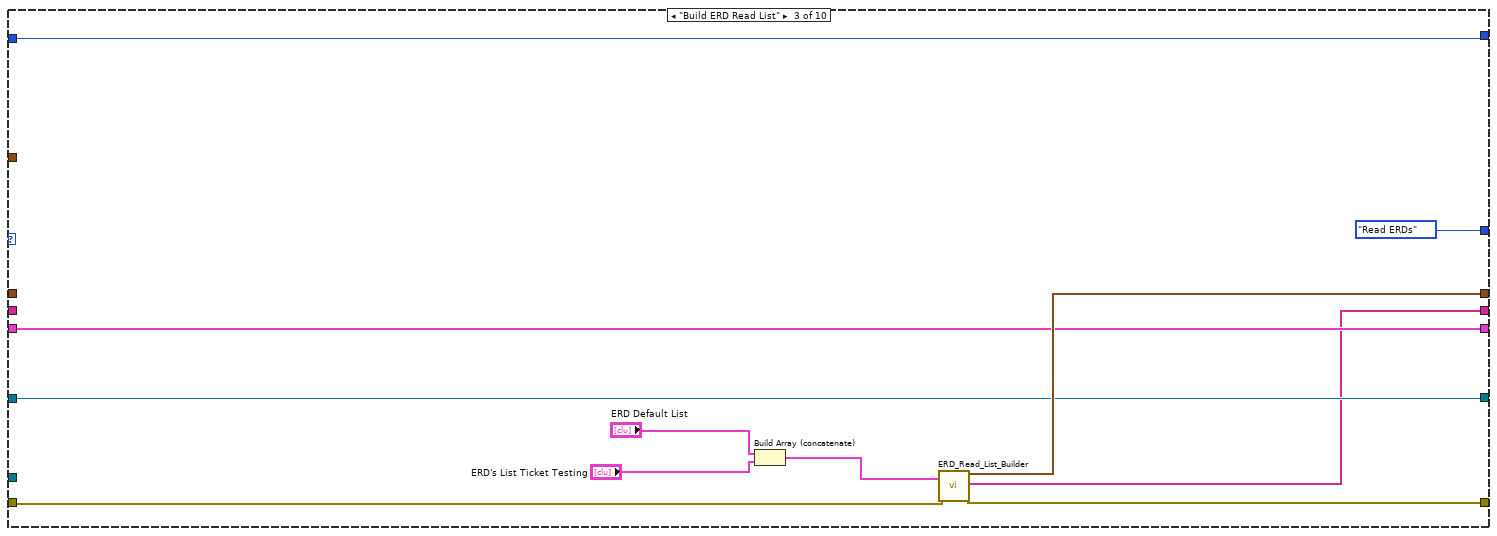
[diagram p5: hidden frame]
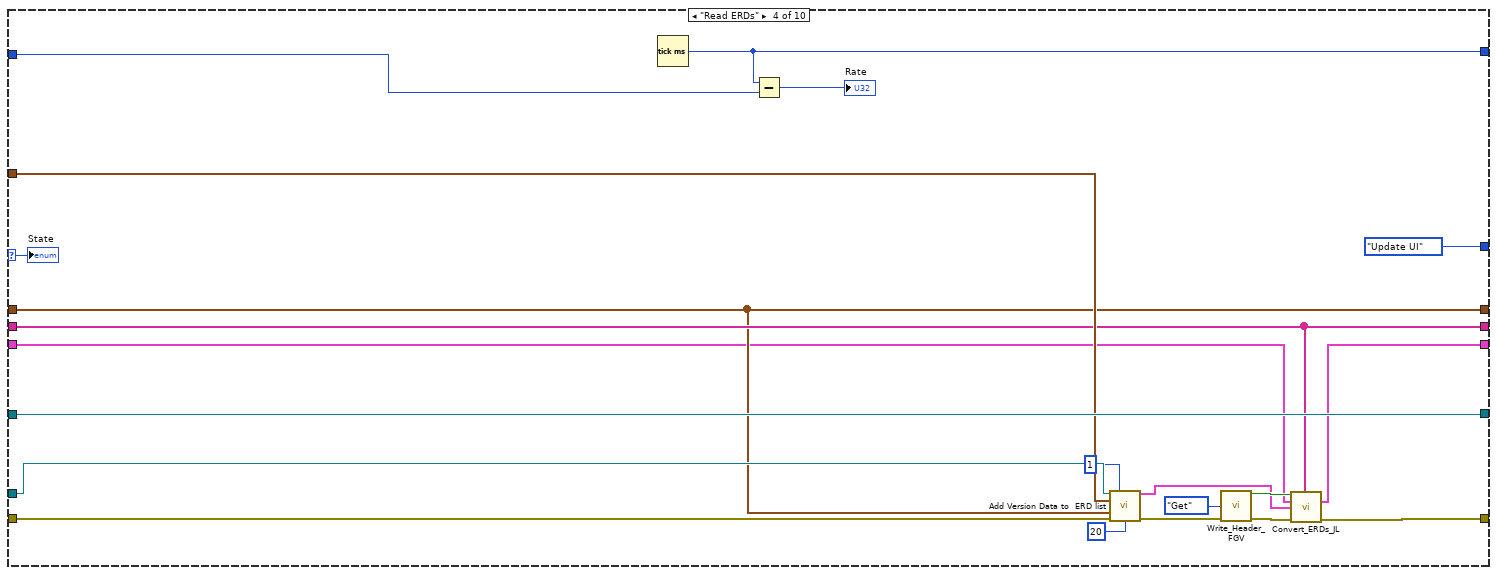
[diagram p6: hidden frame]
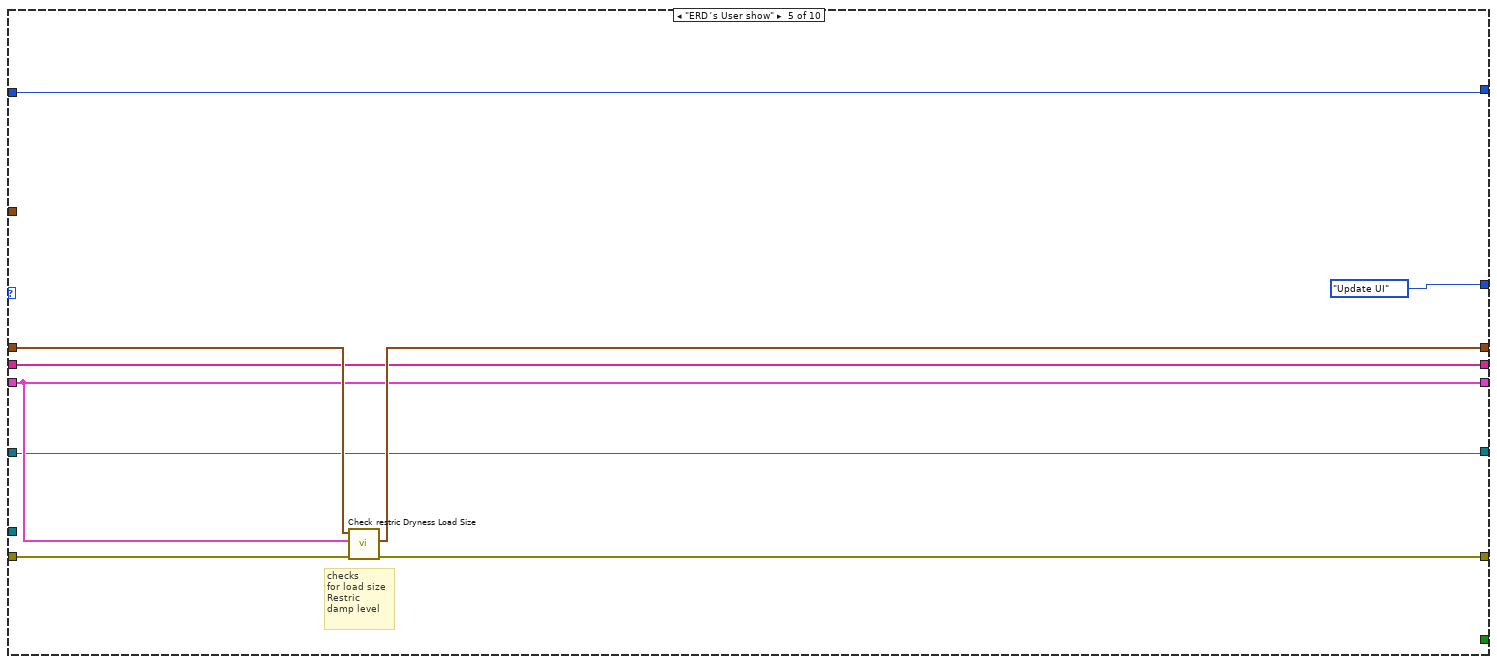
[diagram p7: hidden frame]
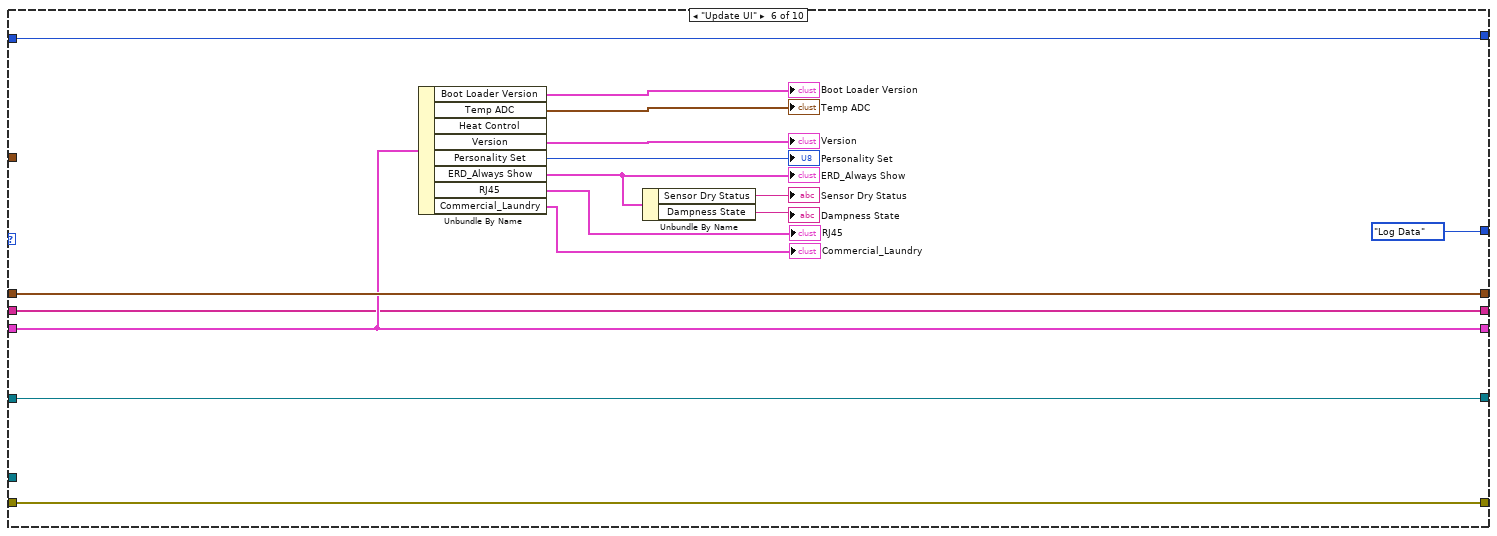
[diagram p8: hidden frame]
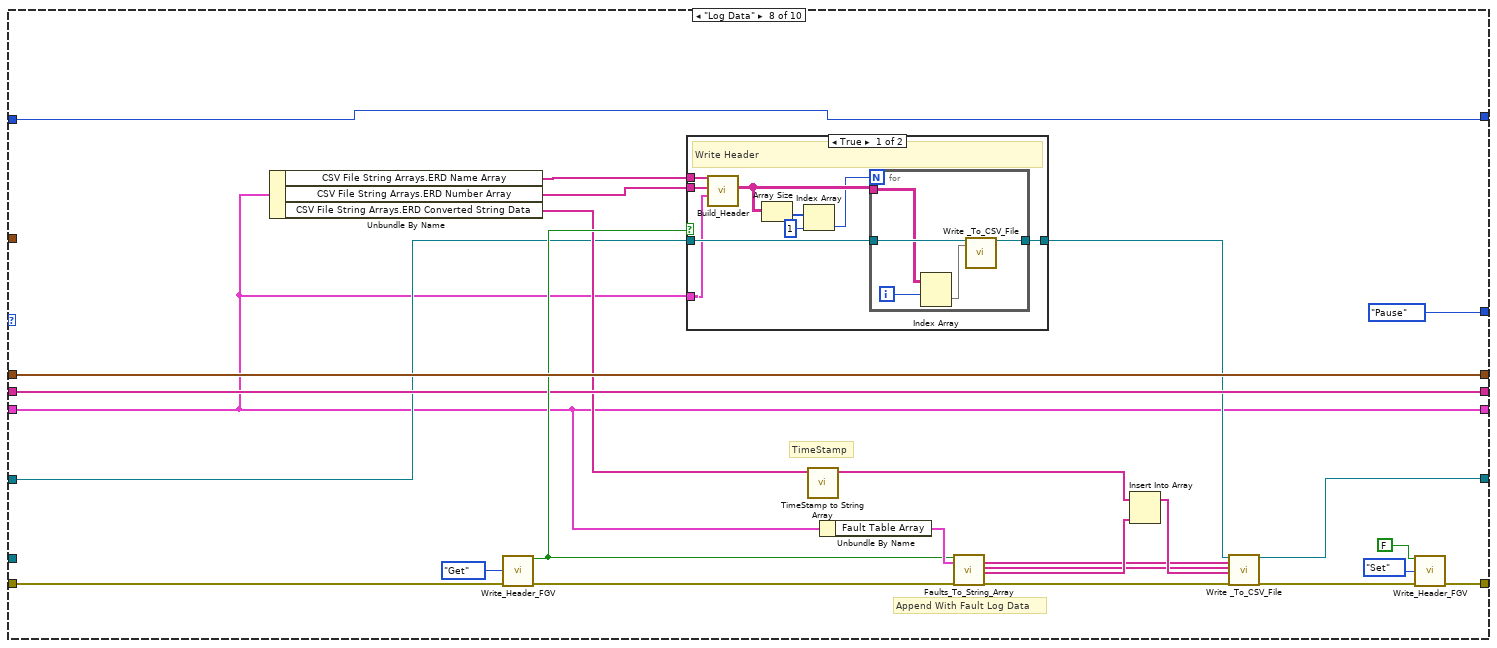
[diagram p9: hidden frame]
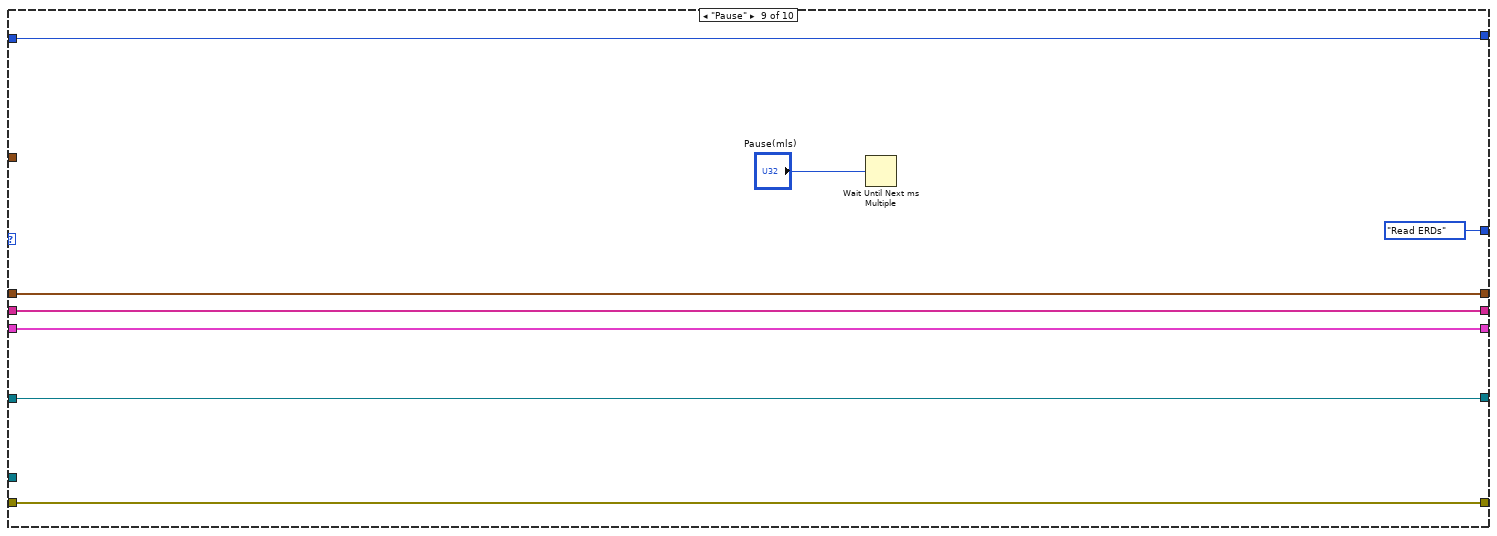
[diagram p11: hidden frame]
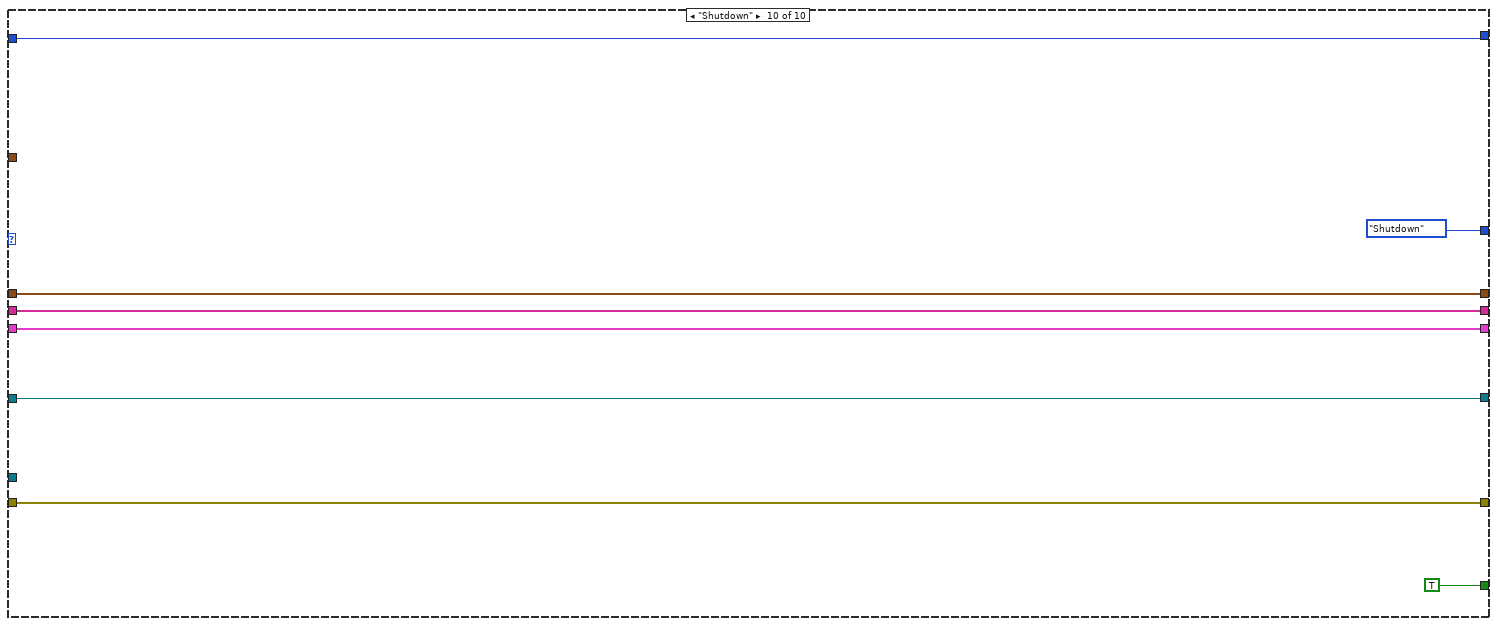
[diagram p12: hidden frame]
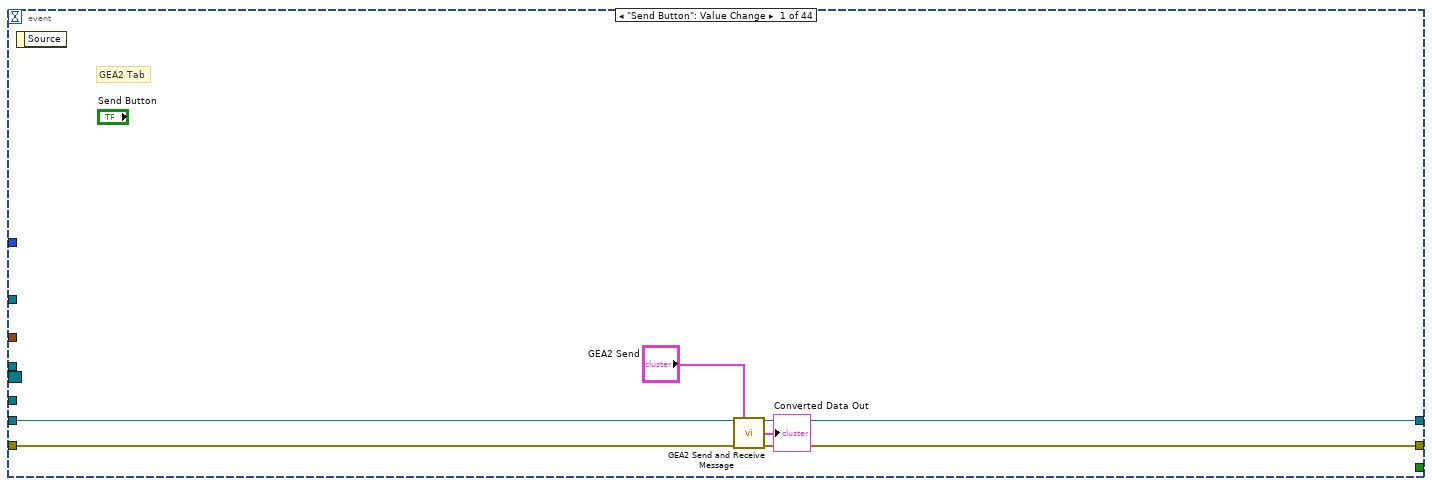
[diagram p13: hidden frame]
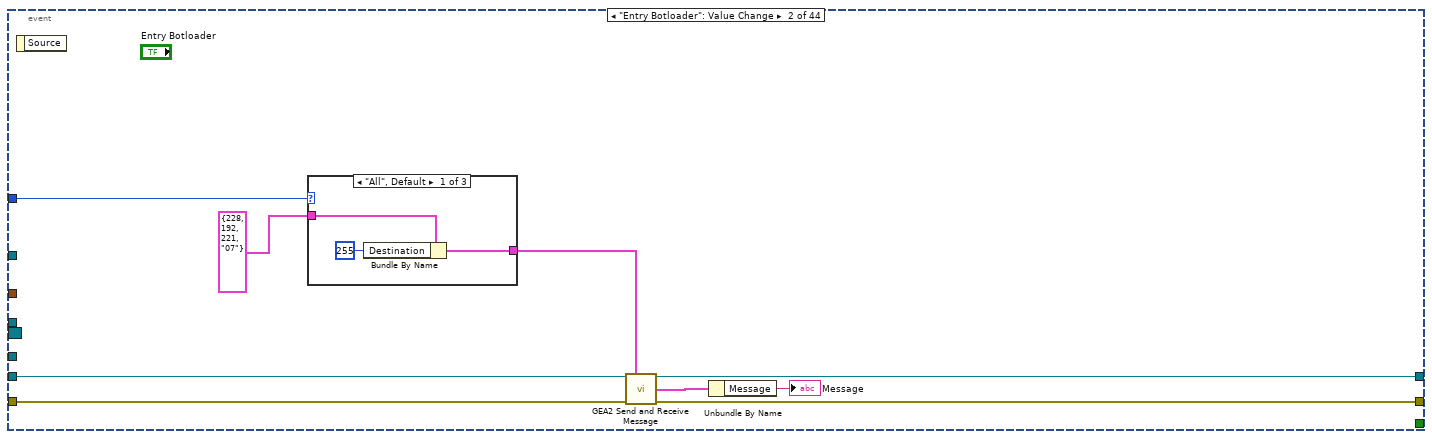
[diagram p14: hidden frame]
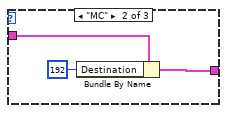
[diagram p15: hidden frame]
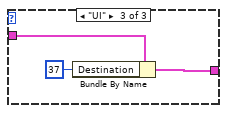
[diagram p16: hidden frame]
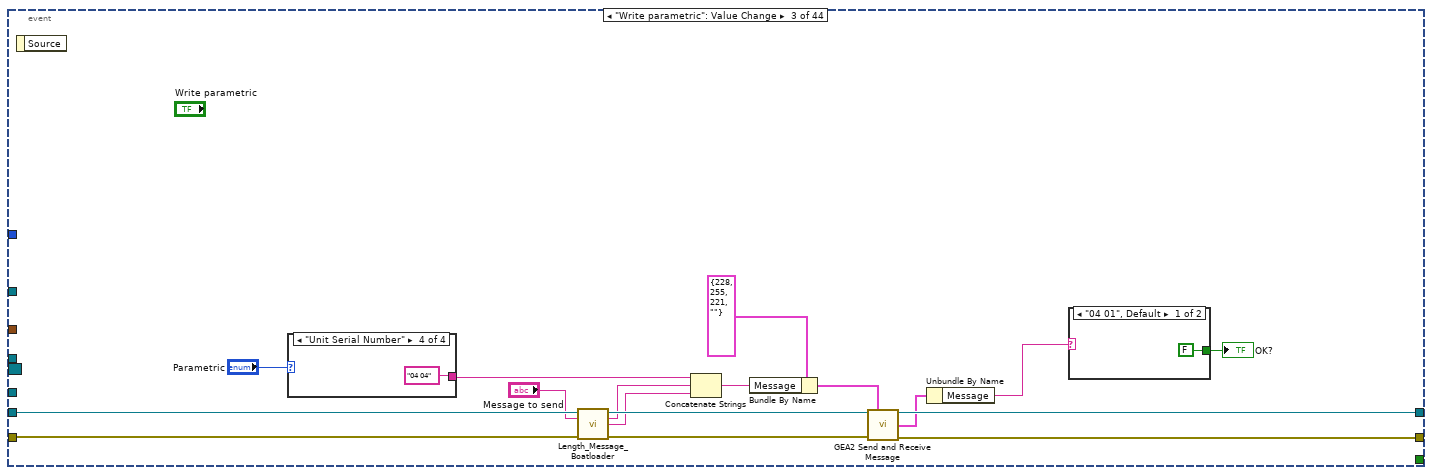
[diagram p17: hidden frame]
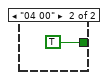
[diagram p18: hidden frame]
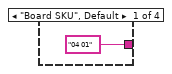
[diagram p19: hidden frame]
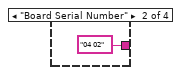
[diagram p20: hidden frame]
diagram:
  # "Get number of NewFIs connected\nand set this to the max value"
  n1 = call "Get NEW FI Set Max.vi"() -> ("Error Out"=w8:errorcluster, "Get Max_Out"=w9:dbl)  [unwired: 10 in]
  n2 = property on="Board Index" class="DigNum (strict)"(error in=w8, "Minimum"=w9) -> (error out=w7:errorcluster)  [unwired: 1 in, 1 out]
  n3 = call "GEA2 Initialize.vi"("Board Index"="Board Index", "Source Address"=u8 229, "error in"=w7) -> ("GEA2 Reference Out"=w5:refnum<k24>, "error out"=w2:errorcluster)  [unwired: 10 in, 1 out]
  n4 = invoke class="GeaNode" method="RegisterAddress"(reference=w5, error in=w2, "address"=u8 229 ("Source Address")) -> (reference out=w3:refnum<k24>, error out=w4:errorcluster)  [unwired: 1 in, 2 out]
  n5 = case shown="No Error" w4 {
    selector: w4 -> [w54 w1235]
    tunnel: [w55 w1235] -> w12
    tunnel: w3 -> [w33 _]
    frame No Error {
      w15 = T22 {"Source"=0, "Destination"=0, "Command"=0, "Length"=0, "CRC"=0, "Message"=""}  # Data_Recv
      w17 = T22 {"Source"=0, "Destination"=0, "Command"=0, "Length"=0, "CRC"=0, "Message"=""}  # Data_Recv
      w25 = errorcluster {"status"=FALSE, "code"=0, "source"=""}  # Receive Loop Error
      # "Se debe dejar el Init pra aejecuete todo los pasos"
      # "store user event in functional\nglobal variable, this will be used\nin the HEUI VI to obtain the proper\nuser event reference"
      # "Store initial GEA2 reference"
      n6 = call "FGV_GEA2_Ref.vi"("GEA2 Reference In"=w33, "Action"=enum16{"Set Ref", "Get Ref"}."Set Ref", "Error In"=w54) -> ("GEA2 Reference Out"=w28:refnum<k24>, "Error Out"=w16:errorcluster)  [unwired: 11 in]
      n7 = vi-ref "GEA2_Toolkit.lvlib:GEA2 Message Received Event Handler.vi"() -> (w26:refnum<vi>)
      n8 = vi-ref "GEA2_Toolkit.lvlib:GEA2 Message Received Event Handler.vi"() -> (w27:refnum<vi>)
      n9 = Create User Event(user event datatype=w17, error in=w16) -> (user event=w21:refnum<user-event>, error out=w30:errorcluster)
      n10 = node(w30, w28, w27, w21) -> (w31:errorcluster)  [unwired: 1 in, 1 out]
      n11 = Create User Event(user event datatype=w15, error in=w31) -> (user event=w22:refnum<user-event>, error out=w29:errorcluster)
      n12 = node(w29, w28, w26, w22) -> (w24:errorcluster)  [unwired: 1 in, 1 out]
      n13 = Create User Event(user event datatype=w25, error in=w24) -> (user event=w18:refnum<user-event>, error out=w23:errorcluster)
      n14 = register-events(error in=w23, w21, w22, w18) -> (reference out=w20:refnum<event-registration>, error out=w19:errorcluster)  [unwired: 1 in]
      n15 = call "UI Loop Error and Que Setup.vi"("error in (no error)"=w19, "Receive Loop"=w18) -> ("error out"=w34:errorcluster, "UI Loop Event Registration"=w32:refnum<event-registration>, "ERD Queue Loop"=w35:refnum<queue>)  [unwired: 6 in, 1 out]
      n16 = call "Get User Filename and Path.vi"("error in (no error)"=w34) -> ("error out"=w36:errorcluster, "CSV File Path"=w38:path)  [unwired: 8 in, 1 out]
      n17 = Create User Event(user event datatype=TRUE ("Bool"), error in=w34) -> (user event=w49:refnum<user-event>, error out=w50:errorcluster)
      n18 = call "Open_Create__Log_File.vi"("File Path Control"=w38, "Enum"=enum16{"CSV File", "Text File"}."CSV File", "Error In"=w36) -> ("refnum out"=w43:refnum<file>, "File Path"=→"CSV File Log Path":path, "Error Out"=w52:errorcluster)  [unwired: 10 in]
      n19 = call "HEUI_Event_FGV.vi"("Event In"=w49, "Action"=enum16{"Get", "Set"}."Set", "Error In"=w50) -> ("Event Out"=w46:refnum<user-event>, "Error Out"=w47:errorcluster)  [unwired: 11 in]
      n20 = Unbundle By Name(T42 {"Data"=variant, "State"=enum."Init"} ("Data")) -> ("State"=w44:T1)
      n21 = while "Periodic ERD Query Loop" {
        shift-right: [w88] -> w42
        shift-left: w52 -> [w90]
        tunnel: w35 -> [w91]
        shift-right: [w82] -> _
        shift-left: w44 -> [w84]
        shift-right: [w77] -> _
        shift-left: _ -> [w76]
        tunnel: w43 -> [w75]
        tunnel: [w74] -> w40
        shift-right: [w73] -> _
        shift-left: T37 {"Version"={"Build Number"="", "Build Hash "="", "Application Version"="", "Parametric Version"="", "UI App Version"=""}, "ERD_Always Show"={"Inlet Thermistor"=0, "Machine State"="", "Filtered Moisture"=0, "Cycle Selected"="", "HTR 1 / Inner / Top"=FALSE, "HTR 2 / Outer / Bot"=FALSE, "Door Switch"=FALSE, "Drum Light"=FALSE, "Cycle Engine State"="", "Centrifugal Switch"=FALSE, "Drum Motor"=FALSE, "Cycle Count"=0, "Ext. Tumble"=FALSE, "eDry"=FALSE, "Temp Level"="", "Dryness Level"="", "Time Level"="", "Delay Time (min)"=0, "Steam Refresh"=FALSE, "Damp Alert"=FALSE, "Sub-Cycle"="", "Outlet Thermistor"=0, "Target Moisture"=0, "Remaining Cycle Time"=0, "Raw Moisture"=0, "Cycle Name"="", "My Cycle"=FALSE, "Delay Dry"=FALSE, "Detangle"=FALSE, "Control Lock"=FALSE, "Steam Valve"=FALSE, "Door Latch"=FALSE, "Signal Volume"="", "Tune ID"="", "Restr Detect Status"="", "Vent Restriction"="", "Load Size by Contact"="", "Load Size by Temp"="", "EOC Reason"="", "Sensor Dry Status"="", "Dampness State"="", "Target Voltage Reached"=FALSE, "TrimInhibitR1"=FALSE, "TrimInhibitR2"=FALSE, "TrimBothCoilInhibit"=FALSE, "NormalHeatControl"=FALSE, "HeatControl Request"=FALSE, "Cool Down Status"="", "EcoDryInhibitRelay1"=FALSE, "EcoDryInhibitRelay2"=FALSE, "ReverseDrumInhibitRelay1"=FALSE, "ReverseDrumInhibitRelay2"=FALSE, "OverTempHeaterInhibitRequest"=FALSE, "FallbackHeatControlMethodStatus"=FALSE, "IHC TimeSeconds"=0, "ECT TimeSeconds "=0, "SC Total Drying Time(S')"=0, "TTR Target Voltage (S')"=0, "TCT Drying Time (S's)"=0, "Drum Motor State"=enum."Off", "Load Size by Ag"="", "MaxFIletered Voltage"=0, "Dry Load Detection"="", "Min Sensing Elapse Sec"=0, "Time Multi Sec X100"=0, "Time Adder  Sec"=0, "Temp Multi EcoDry"="", "Temp Multi ExtraLow"="", "Temp Multi Low "="", "Temp Multi Medium"="", "Temp Multi High"="", "SmoothMoisture"=0, "Eco Dry SEL Status"="", "Eco Dry SEL Result"="", "Eco Dry Cont Status"="", "Eco Dry Relay1 Timer"="", "Eco Dry Relay2 Timer "="", "Eco Dry Stage 2 Tans "=0, "WiFiCommissioningPSt"="", "Payment Method"=""}, "Personality Set"=0, "CSV File String Arrays"={"ERD Number Array"=[], "ERD Name Array"=[], "ERD Converted String Data"=[]}, "Fault Table Array "=[], "Heat Control"={"Htr1 InletLowLim"="", "Htr1 InletUpLim"="", "Htr1 OutletLowLim"="", "Htr1 OutletUpLim"="", "Htr1 FallBackON(s)"="", "Htr1 FallBackOFF(s)"="", "Htr1"=FALSE, "Htr2 InletLowLim"="", "Htr2 InletUpLim"="", "Htr2 OutletLowLim"="", "Htr2 OutletUpLim"="", "Htr2 FallBackON(s)"="", "Htr2 FallBackOFF(s)"="", "Htr2"=FALSE}, "Temp ADC"={"Raw ADC Outlet"=0, "Raw ADC Inlet"=0}, "Commercial_Laundry"={"Session"="", "Phase"="", "Appliance Type"="", "Cycle Selected"="", "Platform Type"="", "Retry Signal"="", "Session Ext"="", "Phase Ext"="", "Appliance Type Ext"="", "Cycle Selected Ext"="", "Platform Type Ext"="", "Retry Signal Ext"=""}, "Boot Loader Version"={"UI BL Version"="", "MC BL Version"=""}, "RJ45"={"Write Access Actual"="", "Write Access Request"="", "LockedAtLeastOnce"=""}} ("All_ERD_Data_Bundled_Brass") -> [w72]
        shift-right: [w70] -> _
        shift-left: _ -> [w69]
        shift-right: [w67] -> _
        shift-left: _ -> [w66]
        stop <- w87 stop-if-true
        # "Todas los pasos de esta ciclo se ejecutan una ves al iniciar el programa"
        # "ERD Loop"
        n22 = Dequeue Element(queue=w91, timeout in ms (-1)=0, error in (no error)=w90) -> (element=w79:T42, timed out?=w71:bool, error out=w89:errorcluster)  [unwired: 1 out]
        n23 = Unbundle By Name(w79) -> ("State"=w85:T1)
        n24 = call "FGV_GEA2_Ref.vi"("Action"=enum16{"Set Ref", "Get Ref"}."Get Ref", "Error In"=w89) -> ("GEA2 Reference Out"=w78:refnum<k24>, "Error Out"=w81:errorcluster)  [unwired: 12 in]
        n25 = Select(t=w84, s=w71, f=w85) -> (s? t:f=w83:T1)
        n26 = case shown="\"Read Faults\"" w83 {
          selector: w83 -> [_ _ _ w158 _ _ _ _ _ _]
          tunnel: w81 -> [w102 w110 w150 w161 w180 w192 _ w223 w250 w258]
          tunnel: [w96 w128 w147 w166 w178 w192 _ w220 w250 w258] -> w86
          tunnel: [_ _ _ _ _ _ _ _ _ TRUE] -> w87
          tunnel: "ERD Spam GEA Inputs" -> [_ _ _ w163 _ _ _ _ _ _]
          tunnel: [ERD_Loop_States."Get Version" ("State") ERD_Loop_States."Build ERD Read List" ("State") ERD_Loop_States."Read ERDs" ("State") ERD_Loop_States."Update UI" ("State") ERD_Loop_States."Update UI" ("State") ERD_Loop_States."Log Data" ("State") ERD_Loop_States."Log Data" ("State") ERD_Loop_States."Pause" ("t") ERD_Loop_States."Read ERDs" ("State") ERD_Loop_States."Shutdown" ("State")] -> w82
          tunnel: w78 -> [_ w111 _ w162 _ _ _ _ _ _]
          tunnel: [w100 w133 w149 w159 w177 w195 w200 w227 w248 w255] -> w77
          tunnel: w76 -> [w100 w133 _ w159 w179 w195 w200 w227 w248 w255]
          tunnel: w75 -> [w99 w132 w146 w170 w175 w193 w199 w208 w247 w254]
          tunnel: [w99 w132 w146 w170 w175 w193 w199 w226 w247 w254] -> w74
          tunnel: [T37 {"Version"={"Build Number"="", "Build Hash "="", "Application Version"="", "Parametric Version"="", "UI App Version"=""}, "ERD_Always Show"={"Inlet Thermistor"=0, "Machine State"="", "Filtered Moisture"=0, "Cycle Selected"="", "HTR 1 / Inner / Top"=FALSE, "HTR 2 / Outer / Bot"=FALSE, "Door Switch"=FALSE, "Drum Light"=FALSE, "Cycle Engine State"="", "Centrifugal Switch"=FALSE, "Drum Motor"=FALSE, "Cycle Count"=0, "Ext. Tumble"=FALSE, "eDry"=FALSE, "Temp Level"="", "Dryness Level"="", "Time Level"="", "Delay Time (min)"=0, "Steam Refresh"=FALSE, "Damp Alert"=FALSE, "Sub-Cycle"="", "Outlet Thermistor"=0, "Target Moisture"=0, "Remaining Cycle Time"=0, "Raw Moisture"=0, "Cycle Name"="", "My Cycle"=FALSE, "Delay Dry"=FALSE, "Detangle"=FALSE, "Control Lock"=FALSE, "Steam Valve"=FALSE, "Door Latch"=FALSE, "Signal Volume"="", "Tune ID"="", "Restr Detect Status"="", "Vent Restriction"="", "Load Size by Contact"="", "Load Size by Temp"="", "EOC Reason"="", "Sensor Dry Status"="", "Dampness State"="", "Target Voltage Reached"=FALSE, "TrimInhibitR1"=FALSE, "TrimInhibitR2"=FALSE, "TrimBothCoilInhibit"=FALSE, "NormalHeatControl"=FALSE, "HeatControl Request"=FALSE, "Cool Down Status"="", "EcoDryInhibitRelay1"=FALSE, "EcoDryInhibitRelay2"=FALSE, "ReverseDrumInhibitRelay1"=FALSE, "ReverseDrumInhibitRelay2"=FALSE, "OverTempHeaterInhibitRequest"=FALSE, "FallbackHeatControlMethodStatus"=FALSE, "IHC TimeSeconds"=0, "ECT TimeSeconds "=0, "SC Total Drying Time(S')"=0, "TTR Target Voltage (S')"=0, "TCT Drying Time (S's)"=0, "Drum Motor State"=enum."Off", "Load Size by Ag"="", "MaxFIletered Voltage"=0, "Dry Load Detection"="", "Min Sensing Elapse Sec"=0, "Time Multi Sec X100"=0, "Time Adder  Sec"=0, "Temp Multi EcoDry"="", "Temp Multi ExtraLow"="", "Temp Multi Low "="", "Temp Multi Medium"="", "Temp Multi High"="", "SmoothMoisture"=0, "Eco Dry SEL Status"="", "Eco Dry SEL Result"="", "Eco Dry Cont Status"="", "Eco Dry Relay1 Timer"="", "Eco Dry Relay2 Timer "="", "Eco Dry Stage 2 Tans "=0, "WiFiCommissioningPSt"="", "Payment Method"=""}, "Personality Set"=0, "CSV File String Arrays"={"ERD Number Array"=[], "ERD Name Array"=[], "ERD Converted String Data"=[]}, "Fault Table Array "=[], "Heat Control"={"Htr1 InletLowLim"="", "Htr1 InletUpLim"="", "Htr1 OutletLowLim"="", "Htr1 OutletUpLim"="", "Htr1 FallBackON(s)"="", "Htr1 FallBackOFF(s)"="", "Htr1"=FALSE, "Htr2 InletLowLim"="", "Htr2 InletUpLim"="", "Htr2 OutletLowLim"="", "Htr2 OutletUpLim"="", "Htr2 FallBackON(s)"="", "Htr2 FallBackOFF(s)"="", "Htr2"=FALSE}, "Temp ADC"={"Raw ADC Outlet"=0, "Raw ADC Inlet"=0}, "Commercial_Laundry"={"Session"="", "Phase"="", "Appliance Type"="", "Cycle Selected"="", "Platform Type"="", "Retry Signal"="", "Session Ext"="", "Phase Ext"="", "Appliance Type Ext"="", "Cycle Selected Ext"="", "Platform Type Ext"="", "Retry Signal Ext"=""}, "Boot Loader Version"={"UI BL Version"="", "MC BL Version"=""}, "RJ45"={"Write Access Actual"="", "Write Access Request"="", "LockedAtLeastOnce"=""}} ("All_ERD_Data_Bundled_Brass") w129 w145 w153 w176 w194 _ w206 w246 w253] -> w73
          tunnel: w72 -> [_ w112 w145 w154 w176 w194 _ w206 w246 w253]
          tunnel: [w95 w114 w144 w160 w173 w187 w198 w211 w245 w252] -> w70
          tunnel: w69 -> [w95 w114 _ w160 w173 w187 w198 w211 w245 w252]
          tunnel: [w94 w131 w143 w157 w172 w186 w197 w210 w244 w251] -> w67
          tunnel: w66 -> [w94 w131 w143 w156 w172 w186 w197 w210 w244 w251]
          frame "Init", Default {
            # "Set Write Header\nFGV to True"
            n27 = call "Write_Header_FGV.vi"("Write Header ? In"=TRUE, "Action"=enum16{"Get", "Set"}."Set", "Error In"=w102) -> ("Error Out"=w96:errorcluster)  [unwired: 11 in, 1 out]
          }
          frame "Get Version" {
            w119 = T8[] [{"ERD Number"=57, "Data Type"=enum."string"}, {"ERD Number"=58, "Data Type"=enum."string"}]  # Read ERD List MC
            n28 = call "GEA3 Read ERD (Rev 2 API) Multiple Messages.vi"("GEA2 Reference In"=w111, "Retry Count"=1 ("# of Iterations (Should be 2 except JL)"), "Read Timeout (ms)"=u32 250, "GEA Inputs"=cluster{"Source":u8, "Destination":u8} {"Source"=229, "Destination"=37}, "Read ERD List"=w119, "Error In"=w110, "Verify ERD Response?"=FALSE) -> ("GEA2 Reference Out"=w106:refnum<k24>, "ERD Data Out"=w115:cluster{"ERD Number":u16, "Data":string}[], "Error Out"=w117:errorcluster)  [unwired: 5 in, 1 out]
            n29 = call "Convert_UI_ERD.vi"("New Header?"=TRUE, "ERD Name"=w114, "ERD_Data_Bundled_Out"=w112, "Array"=w115, "Error In"=w117) -> ("All_ERD_Data_Bundled_Brass"=w104:T37, "Error Out"=w108:errorcluster)  [unwired: 9 in]
            n30 = case shown="True" TRUE {
              tunnel: [w135 w139] -> w109
              tunnel: w108 -> [w135 w139]
              tunnel: [w136 w138] -> w107
              tunnel: w106 -> [w136 w138]
              frame False {
              }
              frame True {
                n31 = Wait Until Next ms Multiple(millisecond multiple=u32 100) -> ()  [unwired: 1 out]
              }
            }
            n32 = call "GEA3 Read ERD (Rev 2 API) Multiple Messages.vi"("GEA2 Reference In"=w107, "Retry Count"=1 ("# of Iterations (Should be 2 except JL)"), "Read Timeout (ms)"=u32 250, "GEA Inputs"=cluster{"Source":u8, "Destination":u8} {"Source"=229, "Destination"=192}, "Read ERD List"=T8[] [{"ERD Number"=127, "Data Type"=enum."string"}, {"ERD Number"=49, "Data Type"=enum."string"}, {"ERD Number"=59, "Data Type"=enum."string"}] ("Read ERD List MC"), "Error In"=w109, "Verify ERD Response?"=FALSE) -> ("ERD Data Out"=w116:cluster{"ERD Number":u16, "Data":string}[], "Error Out"=w125:errorcluster)  [unwired: 5 in, 2 out]
            n33 = call "Convert_ERDs_JL.vi"("New Header?"=TRUE, "ERD Name"=w114, "ERD_Data_Bundled_Out"=w104, "Array"=w116, "Error In"=w125) -> ("All_ERD_Data_Bundled_Brass"=w129:T37, "Error Out"=w128:errorcluster)  [unwired: 9 in]
          }
          frame "Build ERD Read List" {
            n34 = Build Array (concatenate)("ERD Default List", "ERD's List Ticket Testing") -> (w141:T35)
            n35 = call "ERD_Read_List_Builder.vi"("ERD Read List ALL"=w141, "Error In"=w150) -> ("Read ERD List"=w149:T8[], "ERD Name"=w144:string[], "Error Out"=w147:errorcluster)  [unwired: 15 in]
          }
          frame "Read ERDs" {
            n36 = Tick Count (ms)() -> (millisecond timer value=w157:u32)
            n37 = Subtract(x=w157, y=w156) -> (x-y=→"Rate":u32)
            n38 = call "Add Version Data to  ERD list.vi"(".NET Refnum in"=w162, "# of Iterations (Should be 2 except JL)"=1, "GEA Inputs"=w163, "Read ERD List MC"=w159, "error in (no error)"=w161, "#ERDs per message"=20) -> ("ERD Data Out out"=w165:T11[], "error out"=w164:errorcluster)  [unwired: 8 in]
            n39 = call "Write_Header_FGV.vi"("Action"=enum16{"Get", "Set"}."Get", "Error In"=w164) -> ("Write Header ? Out"=w167:bool, "Error Out"=w169:errorcluster)  [unwired: 12 in]
            n40 = call "Convert_ERDs_JL.vi"("New Header?"=w167, "ERD Name"=w160, "ERD_Data_Bundled_Out"=w154, "Array"=w165, "Error In"=w169) -> ("All_ERD_Data_Bundled_Brass"=w153:T37, "Error Out"=w166:errorcluster)  [unwired: 9 in]
            "State" <- w158
          }
          frame "ERD´s User show" {
            # "checks \nfor load size \nRestric\ndamp level"
            n41 = call "Check restric Dryness Load Size.vi"("Error In"=w180, "All_ERD_Data_Bundled_Brass out"=w176, "Read ERD List"=w179) -> ("Error Out"=w178:errorcluster, "New ERD Data"=w177:T8[])  [unwired: 7 in]
          }
          frame "Update UI" {
            n42 = Unbundle By Name(w194) -> ("Boot Loader Version"=→"Boot Loader Version":T12, "Temp ADC"=→"Temp ADC":T3, "Version"=→"Version":T7, "Personality Set"=→"Personality Set":u8, "ERD_Always Show"=w191:T2, "RJ45"=→"RJ45":T6, "Commercial_Laundry"=→"Commercial_Laundry":T5)  [unwired: 1 out]
            "ERD_Always Show" <- w191
            n43 = Unbundle By Name(w191) -> ("Sensor Dry Status"=→"Sensor Dry Status":string, "Dampness State"=→"Dampness State":string)
          }
          frame "Read Faults" {
          }
          frame "Log Data" {
            # "TimeStamp"
            # "Append With Fault Log Data"
            n44 = Unbundle By Name(w206) -> ("CSV File String Arrays.ERD Name Array"=w225:string[], "CSV File String Arrays.ERD Number Array"=w202:string[], "CSV File String Arrays.ERD Converted String Data"=w209:string[])
            n45 = call "Write_Header_FGV.vi"("Action"=enum16{"Get", "Set"}."Get", "Error In"=w223) -> ("Write Header ? Out"=w212:bool, "Error Out"=w218:errorcluster)  [unwired: 12 in]
            n46 = case shown="True" w212 {
              tunnel: w225 -> [w236 _]
              tunnel: w208 -> [w235 w242]
              tunnel: [w234 w242] -> w207
              tunnel: w206 -> [w233 _]
              tunnel: w202 -> [w232 _]
              frame True {
                # "Write Header"
                n47 = call "Build_Header.vi"("All_ERD_Data_Bundled_Brass out"=w233, "ERD Number Array In"=w232, "ERD Name Array In"=w236) -> ("ERD Name Array out 2"=w231:string[][])  [unwired: 8 in]
                n48 = Array Size(array=w231) -> (size(s)=w230:i32[])
                n49 = Index Array(array=w230, index=1) -> (element=w228:i32)
                n50 = for {
                  N: w228 -> [_]
                  tunnel: w235 -> [w241]
                  tunnel: [w240] -> w234
                  tunnel: w231 -> [w239]
                  i -> [w238]
                  n51 = Index Array(array=w239, index (row)=w238) -> (element=w237:string[])  [unwired: 1 in]
                  n52 = call "Write _To_CSV_File.vi"("Refnum In"=w241, "ERD Name"=w237) -> ("Refnum Out"=w240:refnum<file>)  [unwired: 15 in, 2 out]
                }
              }
              frame False {
              }
            }
            n53 = call "TimeStamp to String Array.vi"("String Array In"=w209) -> ("String Array Out"=w205:string[])  [unwired: 10 in]
            n54 = Unbundle By Name(w206) -> ("Fault Table Array"=w214:T39)
            n55 = call "Faults_To_String_Array.vi"("Write Header ?"=w212, "Fault Table Entry"=w214, "Error In"=w218) -> ("Fault Header String Array"=w204:string[], "Fault ERD Number String Array"=w203:string[], "Fault Data String Array"=w217:string[], "Error Out"=w215:errorcluster)  [unwired: 13 in]
            n56 = Insert Into Array(array=w205, new element=w217) -> (w216:string[])  [unwired: 1 in]
            n57 = call "Write _To_CSV_File.vi"("Refnum In"=w207, "ERD Name"=w204, "ERD Number"=w203, "ERD Data"=w216, "Error In"=w215) -> ("Refnum Out"=w226:refnum<file>, "Error Out"=w221:errorcluster)  [unwired: 12 in, 1 out]
            n58 = call "Write_Header_FGV.vi"("Write Header ? In"=FALSE, "Action"=enum16{"Get", "Set"}."Set", "Error In"=w221) -> ("Error Out"=w220:errorcluster)  [unwired: 11 in, 1 out]
          }
          frame "Pause" {
            n59 = Wait Until Next ms Multiple(millisecond multiple="Pause(mls)") -> ()  [unwired: 1 out]
          }
          frame "Shutdown" {
          }
        }
        n60 = call "Error_Control.vi"("Error In"=w86) -> ("Error Out"=w88:errorcluster)  [unwired: 14 in]
      }
      n61 = while "UI Loop" {
        shift-right: [w271] -> w65
        shift-left: w47 -> [w265]
        shift-right: [w273] -> w64
        shift-left: _ -> [_]
        tunnel: w32 -> [w272]
        tunnel: w46 -> [w262]
        tunnel: w35 -> [w261]
        tunnel: w20 -> [w260]
        stop <- w270 stop-if-true
        # "UI Loop"
        n62 = call "FGV_GEA2_Ref.vi"("Action"=enum16{"Set Ref", "Get Ref"}."Get Ref", "Error In"=w265) -> ("GEA2 Reference Out"=w264:refnum<k24>, "Error Out"=w266:errorcluster)  [unwired: 12 in]
        n63 = event shown="[19] \"Run Script\": Value Change" {
          selector: w272 -> [_ _ _ _ _ _ _ _ _ _ _ _ _ _ _ _ _ _ _ _ _ _ _ _ _ _ _ _ _ _ _ _ _ _ _ _ _ _ _ _ _ _ _ _]
          dyn-events: _ -> [_ _ _ _ _ _ _ _ _ _ _ _ _ _ _ _ _ _ _ _ _ _ _ _ _ _ _ _ _ _ _ _ _ _ _ _ _ _ _ _ _ _ _ _]
          timeout: 50 -> [_ _ _ _ _ _ _ _ _ _ _ _ _ _ _ _ _ _ _ _ _ _ _ _ _ _ _ _ _ _ _ _ _ _ _ _ _ _ _ _ _ _ _ _]
          tunnel: [w276 w285 w312 w321 w342 w348 w360 w364 w381 w384 w399 w412 w425 w468 w521 w527 w542 w599 w640 w648 w692 w782 w862 w869 w884 w916 w932 w960 w971 w984 w995 w1007 w1028 w1035 w1049 w1067 _ w1129 w1136 w1170 w1175 w1199 w1212 w1225] -> w269
          tunnel: w266 -> [w277 w287 w305 w324 w339 w346 w360 w365 w376 w383 w398 w419 w433 w473 w526 w537 w544 w601 w638 w645 w694 w784 w860 w870 w885 w917 w929 w961 w979 w984 w1002 w1015 w1027 w1040 w1058 w1070 w1086 w1133 w1138 w1172 w1179 w1195 w1216 w1223]
          tunnel: [_ _ _ _ _ _ _ _ _ _ _ _ _ _ _ _ _ _ _ _ _ _ _ _ _ _ _ _ TRUE _ _ _ _ _ _ _ _ _ _ _ _ _ _ _] -> w270
          tunnel: w264 -> [w278 w288 w311 w323 w341 w352 w361 w368 w378 w387 _ w418 w434 w474 w525 w536 w540 w598 w636 w657 w695 w785 _ w867 w882 w920 w930 _ w982 w985 w1001 w1016 w1032 w1038 w1055 w1069 w1087 w1134 w1137 w1173 w1178 w1196 w1217 w1224]
          tunnel: [w279 w286 w313 w322 w341 _ w361 w369 w382 w388 _ w417 _ _ _ w535 w539 w597 w634 _ w691 w781 _ w868 w883 w918 w931 _ w982 w985 w996 w1005 w1029 w1034 w1050 w1066 _ w1130 w1135 w1171 w1176 w1200 w1213 w1226] -> w273
          tunnel: "GEA Inputs" -> [_ _ _ _ _ w351 _ w367 w377 w386 _ w416 _ _ _ _ w538 w596 w635 _ w696 w786 _ w866 w886 w919 w933 _ _ _ _ w1004 w1017 w1033 w1054 w1068 w1088 w1131 _ w1169 w1177 w1182 w1211 w1222]
          tunnel: w262 -> [_ _ _ _ _ _ _ _ _ _ _ _ w430 w472 _ _ _ _ _ w642 _ _ _ _ _ _ _ _ _ _ _ _ _ _ _ _ _ _ _ _ _ _ _ _]
          tunnel: w261 -> [_ _ _ _ _ w347 _ _ _ _ _ _ w424 w469 w520 _ _ _ w639 w643 _ _ w858 _ _ _ _ w958 w970 _ _ _ _ _ _ _ _ _ _ _ _ _ _ _]
          tunnel: w260 -> [_ _ _ _ _ _ _ _ _ _ _ _ _ _ _ _ _ _ _ _ _ _ _ _ _ _ _ _ _ _ _ _ _ _ _ _ _ _ _ _ _ _ _ _]
          tunnel: "Enum" -> [_ w280 _ w320 _ _ _ _ _ _ _ _ _ _ _ _ _ _ _ _ _ _ _ _ _ _ _ _ _ _ _ _ _ _ _ _ _ _ _ _ _ _ _ _]
          event "Send Button": Value Change {
            # "GEA2 Tab"
            n64 = event-data() -> ()  [unwired: 1 in, 1 out]
            n65 = call "GEA2 Send and Receive Message.vi"("GEA2 Reference In"=w278, "Input Data"="GEA2 Send", "Error In"=w277) -> ("GEA2 Reference Out"=w279:refnum<k24>, "Converted Data Out"=→"Converted Data Out":T22, "Error Out"=w276:errorcluster)  [unwired: 9 in, 1 out]
          }
          event "Entry Botloader": Value Change {
            n66 = event-data() -> ()  [unwired: 1 in, 1 out]
            n67 = case shown="\"All\", Default" w280 {
              tunnel: T21 {"Source"=228, "Destination"=192, "Command"=221, "Message"="07"} ("GEA2 Send") -> [w290 w294 w295]
              tunnel: [w289 w292 w296] -> w281
              frame "All", Default {
                n68 = Bundle By Name(cluster=w290, "Destination"=u8 255) -> (w289:T21)
              }
              frame "MC" {
                n69 = Bundle By Name(cluster=w294, "Destination"=u8 192) -> (w292:T21)
              }
              frame "UI" {
                n70 = Bundle By Name(cluster=w295, "Destination"=u8 37) -> (w296:T21)
              }
            }
            n71 = call "GEA2 Send and Receive Message.vi"("GEA2 Reference In"=w288, "Input Data"=w281, "Error In"=w287) -> ("GEA2 Reference Out"=w286:refnum<k24>, "Converted Data Out"=w284:T22, "Error Out"=w285:errorcluster)  [unwired: 9 in, 1 out]
            n72 = Unbundle By Name(w284) -> ("Message"=→"Message":string)
          }
          event "Write parametric": Value Change {
            n73 = event-data() -> ()  [unwired: 1 in, 1 out]
            n74 = case shown="\"Unit Serial Number\"" "Parametric" {
              tunnel: ["04 01" ("string") "04 02" ("string") "04 03" ("string") "04 04" ("string")] -> w309
              frame "Board SKU", Default {
              }
              frame "Board Serial Number" {
              }
              frame "Unit SKU" {
              }
              frame "Unit Serial Number" {
              }
            }
            n75 = call "Length_Message_Boatloader.vi"("string"="Message to send", "error in"=w305) -> ("hex integer string"=w307:string, "Message"=w306:string, "error out"=w304:errorcluster)  [unwired: 11 in]
            n76 = Concatenate Strings(w309, w307, w306) -> (w302:string)
            n77 = Bundle By Name(cluster=T21 {"Source"=228, "Destination"=255, "Command"=221, "Message"=""} ("GEA2 Send"), "Message"=w302) -> (w301:T21)
            n78 = call "GEA2 Send and Receive Message.vi"("GEA2 Reference In"=w311, "Input Data"=w301, "Error In"=w304) -> ("GEA2 Reference Out"=w313:refnum<k24>, "Converted Data Out"=w300:T22, "Error Out"=w312:errorcluster)  [unwired: 9 in, 1 out]
            n79 = Unbundle By Name(w300) -> ("Message"=w299:string)
            n80 = case shown="\"04 01\", Default" w299 {
              tunnel: [FALSE TRUE] -> w298
              frame "04 01", Default {
              }
              frame "04 00" {
              }
            }
            "OK?" <- w298
          }
          event "Exit Botloader": Value Change {
            n81 = event-data() -> ()  [unwired: 1 in, 1 out]
            n82 = case shown="\"All\", Default" w320 {
              tunnel: T21 {"Source"=228, "Destination"=0, "Command"=221, "Message"="F4 01"} ("GEA2 Send") -> [w328 w332 w333]
              tunnel: [w327 w330 w334] -> w325
              frame "All", Default {
                n83 = Bundle By Name(cluster=w328, "Destination"=u8 255) -> (w327:T21)
              }
              frame "MC" {
                n84 = Bundle By Name(cluster=w332, "Destination"=u8 192) -> (w330:T21)
              }
              frame "UI" {
                n85 = Bundle By Name(cluster=w333, "Destination"=u8 37) -> (w334:T21)
              }
            }
            n86 = call "GEA2 Send and Receive Message.vi"("GEA2 Reference In"=w323, "Input Data"=w325, "Error In"=w324) -> ("GEA2 Reference Out"=w322:refnum<k24>, "Error Out"=w321:errorcluster)  [unwired: 9 in, 2 out]
          }
          event "Clear": Value Change {
            w336 = T49 {"Data"=variant, "State"=enum."Clear"} ("element")
            # "GEA2 Tab"
            n87 = event-data() -> ()  [unwired: 1 in, 6 out]
            n88 = Obtain Queue(name (unnamed)="GEA2", element data type=w336, error in (no error)=w339) -> (queue out=w337:refnum<queue>, error out=w340:errorcluster)  [unwired: 2 in, 1 out]
            n89 = Enqueue Element(queue=w337, element=w336, error in (no error)=w340) -> (error out=w342:errorcluster)  [unwired: 1 in, 2 out]
          }
          event "Set Personality": Value Change {
            # "GEA2 Tab"
            n90 = event-data() -> ()  [unwired: 1 in, 6 out]
            n91 = Index Array(array=T9[] [{"ERD Number"=65281, "Data Type"=enum."string", "Data"=""}] ("Write ERD List")) -> (element=w357:T9)  [unwired: 1 in]
            n92 = Number To Hexadecimal String(1:i16 2 ("width (-)"), 2:"?") -> (0:w356:string)
            n93 = Bundle By Name(cluster=w357, "Data"=w356) -> (w355:T9)
            n94 = Build Array(w355) -> (w354:T9[])
            n95 = call "GEA2 Write ERD.vi"("GEA2 Reference In"=w352, "GEA Inputs"=w351, "Write ERD List"=w354, "Error In"=w346, "Verify ERD Response?"=TRUE) -> ("Error Out"=w344:errorcluster)  [unwired: 8 in, 2 out]
            n96 = call "Get NEW FI Set Max.vi"("error in (no error)"=w344) -> ("Error Out"=w343:errorcluster)  [unwired: 9 in, 1 out]
            n97 = call "FGV_GEA2_Ref.vi"("Action"=enum16{"Set Ref", "Get Ref"}."Get Ref", "Error In"=w343) -> ()  [unwired: 12 in, 2 out]
            n98 = Enqueue Element(queue=w347, element=T42 {"Data"=variant, "State"=enum."Init"} ("Data")) -> (error out=w348:errorcluster)  [unwired: 2 in, 2 out]
          }
          event Timeout {
            # "Must have timeout case to give GEA2 FGV a chance to update\nthe GEA2 reference. Otherwise, when we receive an event it may\nbe using a reference that is no longer valid."
            n99 = event-data() -> ()  [unwired: 1 in, 3 out]
          }
          event "Write ERD": Value Change {
            # "Read/Write ERDs Tab"
            n100 = event-data() -> ()  [unwired: 1 in, 1 out]
            n101 = call "GEA3 Write ERD (Rev 2 API) Multiple Messages.vi"("GEA2 Reference In"=w368, "# of Tries"=2 ("Retry Count"), "GEA Inputs"=w367, "Write ERD List"="Write ERD List", "Error In"=w365, "Verify ERD Response?"=TRUE) -> ("GEA2 Reference Out"=w369:refnum<k24>, "Error Out"=w364:errorcluster)  [unwired: 7 in, 1 out]
          }
          event "Enable CC Mode": Value Change {
            # "ERD Controls tab"
            n102 = event-data() -> ()  [unwired: 1 in, 1 out]
            n103 = call "Commercial2_Continuous Cycle Mode Config.vi"("GEA2 Reference In"=w378, "Completed Cycles"="Completed Cycles", "Enabled"="Enabled", "GEA Inputs"=w377, "TimeBetween Cycles"="TimeBetween Cycles", "Requested Cycles"="Requested Cycles", "Error In"=w376) -> ("GEA2 Reference Out"=w371:refnum<k24>, "Error Out"=w370:errorcluster)  [unwired: 6 in, 1 out]
            n104 = call "GEA2 Write ERD.vi"("GEA2 Reference In"=w371, "# of Tries"=2 ("Retry Count"), "GEA Inputs"=w377, "Write ERD List"=T9[] [{"ERD Number"=61770, "Data Type"=enum."string", "Data"="01"}], "Error In"=w370) -> ("GEA2 Reference Out"=w382:refnum<k24>, "Error Out"=w381:errorcluster)  [unwired: 8 in, 1 out]
          }
          event "Read ERD": Value Change {
            # "Read/Write ERDs tab"
            n105 = event-data() -> ()  [unwired: 1 in, 6 out]
            n106 = call "GEA3 Read ERD (Rev 2 API) Multiple Messages.vi"("GEA2 Reference In"=w387, "Retry Count"=2, "GEA Inputs"=w386, "Read ERD List"="Read ERD List", "Error In"=w383, "Verify ERD Response?"=TRUE) -> ("GEA2 Reference Out"=w388:refnum<k24>, "ERD Data Out"=→"Read ERD Data Out":cluster{"ERD Number":u16, "Data":string}[], "Error Out"=w384:errorcluster)  [unwired: 6 in, 1 out]
          }
          event "UI Launch": Value Change {
            # "Main"
            n107 = event-data() -> ()  [unwired: 1 in, 6 out]
            n108 = call "HEUI_Running_FGV.vi"("Action"=enum16{"Get", "Set"}."Get", "Error In"=w398) -> ("Running?"=w395:bool, "Error Out"=w397:errorcluster)  [unwired: 12 in]
            n109 = Current VI's Path() -> (path=w393:path)
            n110 = Strip Path(path=w393) -> (stripped path=w394:path)  [unwired: 1 out]
            n111 = case shown="False" w395 {
              tunnel: w397 -> [w409 w411]
              tunnel: [w408 w411] -> w399
              tunnel: w394 -> [w401 _]
              tunnel: "UI Launch" -> [_ _]
              frame False {
                w410 = 128  # options
                n112 = Build Path(base path=w401, name or relative path="JLMainUI.vi") -> (appended path=w406:path)
                n113 = Open VI Reference(type specifier VI Refnum (for type only)=refnum<vi> refnum, vi path=w406, options=w410, error in (no error)=w409) -> (vi reference=w403:refnum<vi>, error out=w405:errorcluster)  [unwired: 2 in]
                n114 = call-by-ref "Start Asynchronous Call"(reference=w403, error in=w405) -> (reference out=w402:refnum<vi>, error out=w404:errorcluster)  [unwired: 10 in, 2 out]
                n115 = Close Reference(reference=w402, error in (no error)=w404) -> (error out=w408:errorcluster)
              }
              frame True {
              }
            }
          }
          event "Read Parametric": Value Change {
            # "Main"
            n116 = event-data() -> ()  [unwired: 1 in, 6 out]
            n117 = call "Para_ERD_Fxxx.vi"("GEA Inputs"=w416, "Error In"=w419, "Read ERD List"=T8[] [], "GEA2 Reference In"=w418) -> ("Error Out"=w413:errorcluster, "F6XX"=w414:T50, "GEA2 Reference Out"=w417:refnum<k24>)  [unwired: 4 in, 1 out]
            n118 = call "Parametric Viewer.vi"("Error In"=w413, "F6XX_In"=w414) -> ("Error Out"=w412:errorcluster)  [unwired: 8 in, 1 out]
          }
          event Value Change {
            (unwired) "ERD Loop" ("name (unnamed)")
            w426 = TRUE ("Blinking")
            # "GEA2 Tab"
            n119 = event-data() -> ()  [unwired: 1 in, 6 out]
            n120 = Generate User Event(user event=w430, event data cluster=TRUE ("event data"), error in=w433) -> (error out=w431:errorcluster)  [unwired: 1 in, 1 out]
            n121 = property on="Program Ind" class="Bool (strict)"(error in=w431, "Value"=w426, "Blinking"=w426) -> (error out=w427:errorcluster)  [unwired: 1 in, 1 out]
            n122 = Enqueue Element(queue=w424, element=T42 {"Data"=variant, "State"=enum."Pause"} ("Data"), error in (no error)=w427) -> (error out=w429:errorcluster)  [unwired: 1 in, 2 out]
            n123 = property on="GEA2 Send" class="Clust (strict)"() -> ("Value"=w422:T21)  [unwired: 2 in, 2 out]
            n124 = Unbundle By Name("Programming") -> ("File Path"=w437:path)
            n125 = call "Time Delay3"("error in (no error)"=w429, "Delay Time (s)"=2.0) -> ("error out"=w428:errorcluster)  [unwired: 9 in]
            n126 = Unbundle By Name(w422) -> ("Source"=w421:u8, "Destination"=w420:u8)
            n127 = Not Equal?(x=w437, y=path "") -> (x != y?=w436:bool)
            n128 = case shown="True" w436 {
              tunnel: w428 -> [w440 w445]
              tunnel: [w440 w452] -> w425
              tunnel: w437 -> [_ w457]
              tunnel: w434 -> [_ w453]
              tunnel: w421 -> [_ w442]
              tunnel: w420 -> [_ w441]
              frame False {
              }
              frame True {
                w443 = T20 9 items=["ImageRejected", "BoardNotFound", "UnableToGetGeaConfiguration", "WriteToFlashNotAllowed", "ImageDownloadedSuccessfully", "ImagePresent", "WriteToFlashFailed", "EraseFailed", "CrcFailed", ""] ("Result")
                w451 = FALSE ("Blinking")
                n129 = property on="Result" class="Ring (strict)"(error in=w445, "Value"=w443) -> (error out=w444:errorcluster)  [unwired: 1 in, 1 out]
                n130 = property on="Board Index" class="DigNum (strict)"(error in=w445, "DisabledEnum"=T44."Disabled and Grayed Out" ("Disabled")) -> ()  [unwired: 1 in, 2 out]
                n131 = call "GEA2 Flash APL.vi"("GEA2 Reference In"=w453, "Force Update?"=TRUE, "Source Address"=w442, "Destination Address"=w441, "File Path"=w457, "Error In"=w444, "Broadcast"=TRUE, "Reset?"=FALSE ("Reset Board?")) -> ("Result"=w446:i32, "Error Out"=w448:errorcluster)  [unwired: 3 in, 3 out]
                n132 = property on="Result" class="Ring (strict)"(error in=w448, "Value"=w446) -> (error out=w447:errorcluster)  [unwired: 1 in, 1 out]
                n133 = property on="Board Index" class="DigNum (strict)"(error in=w448, "DisabledEnum"=T44."Enabled" ("Disabled")) -> ()  [unwired: 1 in, 2 out]
                n134 = property on="Program Ind" class="Bool (strict)"(error in=w447, "Value"=w451, "Blinking"=w451) -> (error out=w452:errorcluster)  [unwired: 1 in, 1 out]
              }
            }
          }
          event "Flash Latest": Value Change {
            (unwired) "ERD Loop" ("name (unnamed)")
            w463 = TRUE ("Blinking")
            (unwired) FALSE ("Data On")
            # "GEA2 Tab"
            n135 = event-data() -> ()  [unwired: 1 in, 6 out]
            n136 = Generate User Event(user event=w472, event data cluster=TRUE ("event data"), error in=w473) -> (error out=w465:errorcluster)  [unwired: 1 in, 1 out]
            n137 = property on="Program Ind" class="Bool (strict)"(error in=w465, "Value"=w463, "Blinking"=w463) -> (error out=w464:errorcluster)  [unwired: 1 in, 1 out]
            n138 = Enqueue Element(queue=w469, element=T42 {"Data"=variant, "State"=enum."Pause"} ("Data"), error in (no error)=w464) -> (error out=w471:errorcluster)  [unwired: 1 in, 2 out]
            n139 = call "JL_Get_Latest_Build_From_Artifactory.vi"("Repository"="CIBuild") -> ("Output Path"=w458:path)  [unwired: 12 in, 2 out]
            n140 = call "Time Delay2"("error in (no error)"=w471, "Delay Time (s)"=3.0) -> ("error out"=w470:errorcluster)  [unwired: 9 in]
            n141 = Not Equal?(x=w458, y=path "") -> (x != y?=w476:bool)
            n142 = case shown="True" w476 {
              tunnel: w470 -> [w479 w503]
              tunnel: [w479 w491] -> w461
              tunnel: w474 -> [_ w504]
              tunnel: w458 -> [_ w480]
              frame False {
              }
              frame True {
                w483 = T20 9 items=["ImageRejected", "BoardNotFound", "UnableToGetGeaConfiguration", "WriteToFlashNotAllowed", "ImageDownloadedSuccessfully", "ImagePresent", "WriteToFlashFailed", "EraseFailed", "CrcFailed", ""] ("Result")
                w490 = FALSE ("Blinking")
                n143 = call "JL_APLPath.vi"("Error In"=w503, "APL Search String"=T45."UI Application APL", "Folder Path"=w480) -> ("Error Out"=w502:errorcluster, "File Path"=w501:path)  [unwired: 5 in, 2 out]
                n144 = call "GEA2 Flash APL.vi"("GEA2 Reference In"=w504, "Force Update?"=TRUE, "Source Address"=u8 228, "Destination Address"=u8 36, "File Path"=w501, "Error In"=w502, "Broadcast"=TRUE, "Reset?"=FALSE ("Reset Board?")) -> ("GEA2 Reference Out"=w493:refnum<k24>, "Result"=w487:i32, "Error Out"=w489:errorcluster)  [unwired: 3 in, 2 out]
                n145 = property on="Board Index" class="DigNum (strict)"(error in=w503, "DisabledEnum"=T44."Disabled and Grayed Out" ("Disabled")) -> (error out=w486:errorcluster)  [unwired: 1 in, 1 out]
                n146 = property on="Result" class="Ring (strict)"(error in=w489, "Value"=w487) -> (error out=w488:errorcluster)  [unwired: 1 in, 1 out]
                n147 = property on="Result" class="Ring (strict)"(error in=w486, "Value"=w483) -> ()  [unwired: 1 in, 2 out]
                n148 = call "JL_APLPath.vi"("Error In"=w488, "APL Search String"=T45."UI Parametric APL", "Folder Path"=w480) -> ("Error Out"=w499:errorcluster, "File Path"=w500:path)  [unwired: 5 in, 2 out]
                n149 = call "GEA2 Flash APL.vi"("GEA2 Reference In"=w493, "Force Update?"=TRUE, "Source Address"=u8 228, "Destination Address"=u8 36, "File Path"=w500, "Error In"=w499, "Broadcast"=TRUE, "Reset?"=TRUE ("Reset Board?")) -> ("Result"=w484:i32, "Error Out"=w492:errorcluster)  [unwired: 3 in, 3 out]
                n150 = property on="Board Index" class="DigNum (strict)"(error in=w492, "DisabledEnum"=T44."Enabled" ("Disabled")) -> (error out=w485:errorcluster)  [unwired: 1 in, 1 out]
                n151 = property on="Program Ind" class="Bool (strict)"(error in=w492, "Value"=w490, "Blinking"=w490) -> (error out=w491:errorcluster)  [unwired: 1 in, 1 out]
                n152 = property on="Result" class="Ring (strict)"(error in=w485, "Value"=w484) -> ()  [unwired: 1 in, 2 out]
              }
            }
            n153 = call "Time Delay4"("error in (no error)"=w461, "Delay Time (s)"=3.0) -> ("error out"=w460:errorcluster)  [unwired: 9 in]
            n154 = Enqueue Element(queue=w469, element=T42 {"Data"=variant, "State"=enum."Init"} ("Data"), error in (no error)=w460) -> (error out=w468:errorcluster)  [unwired: 1 in, 2 out]
          }
          event Value Change {
            # "GEA2 TAB"
            n155 = event-data() -> ()  [unwired: 1 in, 6 out]
            n156 = property on="GEA2 Send" class="Clust (strict)"() -> ("Value"=w515:T21)  [unwired: 2 in, 2 out]
            n157 = Unbundle By Name(w515) -> ("Source"=w514:u8)
            n158 = Bundle By Name(cluster=T21 {"Source"=228, "Destination"=36, "Command"=221, "Message"="F401"} ("Input Data"), "Source"=w514, "Destination"=u8 255, "Command"=u8 221, "Message"="F401") -> (w518:T21)
            n159 = call "GEA2 Send Message.vi"("GEA2 Reference In"=w525, "Input Data"=w518, "Error In"=w526) -> ("Error Out"=w512:errorcluster)  [unwired: 11 in, 1 out]
            n160 = call "Time Delay5"("error in (no error)"=w512, "Delay Time (s)"=3.0) -> ("error out"=w522:errorcluster)  [unwired: 9 in]
            n161 = Enqueue Element(queue=w520, element=T42 {"Data"=variant, "State"=enum."Init"} ("Data"), error in (no error)=w522) -> (error out=w521:errorcluster)  [unwired: 1 in, 2 out]
          }
          event Value Change {
            # "GEA2 Tab"
            n162 = event-data() -> ()  [unwired: 1 in, 6 out]
            n163 = property on="GEA2 Send" class="Clust (strict)"() -> ("Value"=w534:T21)  [unwired: 2 in, 2 out]
            n164 = Unbundle By Name(w534) -> ("Source"=w530:u8, "Destination"=w529:u8)
            n165 = Bundle By Name(cluster=T21 {"Source"=228, "Destination"=36, "Command"=221, "Message"="F401"} ("Input Data"), "Source"=w530, "Destination"=w529, "Command"=u8 221, "Message"="07") -> (w528:T21)
            n166 = call "GEA2 Send Message.vi"("GEA2 Reference In"=w536, "Input Data"=w528, "Error In"=w537) -> ("GEA2 Reference Out"=w535:refnum<k24>, "Error Out"=w527:errorcluster)  [unwired: 11 in]
          }
          event Value Change {
            # "Load Control Tab"
            n167 = event-data() -> ("CtlRef"=w546:refnum<vi>)  [unwired: 1 in, 5 out]
            n168 = property class="Bool"(reference=w546, error in=w544) -> (error out=w543:errorcluster, "Label.Text"=w545:string)  [unwired: 1 out]
            n169 = case shown="\"Relays ON\"" w545 {
              tunnel: w543 -> [w551 w587]
              tunnel: [w566 w594] -> w542
              tunnel: "Relay Control" -> [w579 _]
              tunnel: w540 -> [w547 w593]
              tunnel: [w561 w589] -> w539
              tunnel: w538 -> [w550 w581]
              frame "Relays ON" {
                n170 = call "GEA2 Write ERD.vi"("GEA2 Reference In"=w547, "GEA Inputs"=w550, "Write ERD List"=T9[] [{"ERD Number"=61795, "Data Type"=enum."string", "Data"="01"}], "Error In"=w551) -> ("Error Out"=w548:errorcluster)  [unwired: 9 in, 2 out]
                n171 = Unbundle By Name(w579) -> ("Drum Motor"=w576:bool, "HTR 1 / Inner / Top"=w571:bool, "HTR 2 / Outer / Bot"=w570:bool, "Steam Valve"=w569:bool, "Pump"=w553:bool)
                n172 = Boolean To (0,1)(Boolean=w576) -> (0, 1=w578:i16)
                n173 = Boolean To (0,1)(Boolean=w571) -> (0, 1=w575:i16)
                n174 = Boolean To (0,1)(Boolean=w570) -> (0, 1=w573:i16)
                n175 = Boolean To (0,1)(Boolean=w569) -> (0, 1=w572:i16)
                n176 = Boolean To (0,1)(Boolean=w553) -> (0, 1=w554:i16)
                n177 = Number To Hexadecimal String(1:i16 2 ("width (-)"), 2:w578) -> (0:w577:string)
                n178 = Number To Hexadecimal String(1:i16 2 ("width (-)"), 2:w575) -> (0:w574:string)
                n179 = Number To Hexadecimal String(1:i16 2 ("width (-)"), 2:w573) -> (0:w568:string)
                n180 = Number To Hexadecimal String(1:i16 2 ("width (-)"), 2:w572) -> (0:w567:string)
                n181 = Number To Hexadecimal String(1:i16 2 ("width (-)"), 2:w554) -> (0:w552:string)
                n182 = Concatenate Strings(w577, w574, w568, w567, w552) -> (w564:string)
                n183 = Bundle By Name(cluster=T9 {"ERD Number"=61457, "Data Type"=enum."string", "Data"=""} ("ERD Read Data In"), "Data"=w564) -> (w563:T9)
                n184 = Build Array(w563) -> (w562:T9[])
                n185 = call "GEA2 Write ERD.vi"("GEA2 Reference In"=w547, "GEA Inputs"=w550, "Write ERD List"=w562, "Error In"=w548, "Verify ERD Response?"=TRUE) -> ("GEA2 Reference Out"=w561:refnum<k24>, "Error Out"=w566:errorcluster)  [unwired: 8 in, 1 out]
              }
              frame "Relays OFF", Default {
                w582 = FALSE ("Value")
                n186 = property on="Drum Motor" class="Bool (strict)"(error in=w587, "Value"=w582) -> (error out=w586:errorcluster)  [unwired: 1 in, 1 out]
                n187 = property on="HTR 1 / Inner / Top" class="Bool (strict)"(error in=w586, "Value"=w582) -> (error out=w585:errorcluster)  [unwired: 1 in, 1 out]
                n188 = property on="HTR 2 / Outer / Bot" class="Bool (strict)"(error in=w585, "Value"=w582) -> (error out=w584:errorcluster)  [unwired: 1 in, 1 out]
                n189 = property on="Steam Valve" class="Bool (strict)"(error in=w584, "Value"=w582) -> (error out=w583:errorcluster)  [unwired: 1 in, 1 out]
                n190 = Bundle By Name(cluster=T9 {"ERD Number"=61457, "Data Type"=enum."string", "Data"=""} ("ERD Read Data In"), "Data"="0000000000") -> (w591:T9)
                n191 = Build Array(w591) -> (w590:T9[])
                n192 = call "GEA2 Write ERD.vi"("GEA2 Reference In"=w593, "GEA Inputs"=w581, "Write ERD List"=w590, "Error In"=w583, "Verify ERD Response?"=TRUE) -> ("GEA2 Reference Out"=w589:refnum<k24>, "Error Out"=w594:errorcluster)  [unwired: 8 in, 1 out]
              }
            }
          }
          event Value Change {
            # "Load Control Tab"
            n193 = event-data() -> ("CtlRef"=w603:refnum<vi>)  [unwired: 1 in, 5 out]
            n194 = property class="Ctl"(reference=w603, error in=w601) -> (error out=w600:errorcluster, "Label.Text"=w602:string)  [unwired: 1 out]
            n195 = case shown="\"Drum Light ON\"" w602 {
              tunnel: w600 -> [w607 w618 w632]
              tunnel: [w610 w617 w631] -> w599
              tunnel: "Drum Light" -> [_ _ w626]
              tunnel: w598 -> [w606 w616 w630]
              tunnel: [w608 w613 w629] -> w597
              tunnel: w596 -> [w604 w612 w628]
              frame "Drum Light ON" {
                n196 = Build Array(T9 {"ERD Number"=61582, "Data Type"=enum."string", "Data"="01"} ("ERD Read Data In")) -> (w605:T9[])
                n197 = call "GEA2 Write ERD.vi"("GEA2 Reference In"=w606, "GEA Inputs"=w604, "Write ERD List"=w605, "Error In"=w607) -> ("GEA2 Reference Out"=w608:refnum<k24>, "Error Out"=w610:errorcluster)  [unwired: 9 in, 1 out]
              }
              frame "Drum Light OFF", Default {
                n198 = Build Array(T9 {"ERD Number"=61582, "Data Type"=enum."string", "Data"="00"} ("ERD Read Data In")) -> (w614:T9[])
                n199 = call "GEA2 Write ERD.vi"("GEA2 Reference In"=w616, "GEA Inputs"=w612, "Write ERD List"=w614, "Error In"=w618, "Verify ERD Response?"=TRUE) -> ("GEA2 Reference Out"=w613:refnum<k24>, "Error Out"=w617:errorcluster)  [unwired: 8 in, 1 out]
              }
              frame "On Time (s)" {
                n200 = Unbundle By Name(w626) -> ("On Time (s)"=w623:dbl)
                n201 = Multiply(x=w623, y=1000.0) -> (x*y=w621:dbl)
                n202 = Number To Decimal String(number=w621) -> (decimal integer string=w620:string)  [unwired: 1 in]
                n203 = Bundle By Name(cluster=T9 {"ERD Number"=61482, "Data Type"=enum."uint32_t", "Data"=""} ("ERD Read Data In"), "Data"=w620) -> (w625:T9)
                n204 = Build Array(w625) -> (w624:T9[])
                n205 = call "GEA2 Write ERD.vi"("GEA2 Reference In"=w630, "GEA Inputs"=w628, "Write ERD List"=w624, "Error In"=w632, "Verify ERD Response?"=TRUE) -> ("GEA2 Reference Out"=w629:refnum<k24>, "Error Out"=w631:errorcluster)  [unwired: 8 in, 1 out]
              }
            }
          }
          event "Reset": Value Change {
            # "Main"
            n206 = event-data() -> ()  [unwired: 1 in, 6 out]
            n207 = call "GEA2 Write ERD.vi"("GEA2 Reference In"=w636, "GEA Inputs"=w635, "Write ERD List"=T9[] [{"ERD Number"=50, "Data Type"=enum."string", "Data"="01"}], "Error In"=w638) -> ("GEA2 Reference Out"=w634:refnum<k24>, "Error Out"=w633:errorcluster)  [unwired: 9 in, 1 out]
            n208 = Enqueue Element(queue=w639, element=T42 {"Data"=variant, "State"=enum."Init"} ("Data"), error in (no error)=w633) -> (error out=w640:errorcluster)  [unwired: 1 in, 2 out]
          }
          event "Run Script": Value Change {
            w669 = T33 {"Overall Script File Progress"=0.0, "Current Script Progress"=0.0, "Script"="", "Test"="", "Elapsed time (s)"=0.0, "Done?"=FALSE}  # Script Info
            w661 = T21 {"Source"=228, "Destination"=35, "Command"=1, "Message"=""}  # Version Query (for log header)
            # "Scripting Tab"
            n209 = event-data() -> ()  [unwired: 1 in, 6 out]
            n210 = Generate User Event(user event=w642, event data cluster=TRUE ("event data"), error in=w645) -> (error out=w646:errorcluster)  [unwired: 1 in, 1 out]
            n211 = Enqueue Element(queue=w643, element=T42 {"Data"=variant, "State"=enum."Pause"} ("Data"), error in (no error)=w646) -> (error out=w644:errorcluster)  [unwired: 1 in, 2 out]
            n212 = Obtain Queue(name (unnamed)="Script_Stop", element data type=FALSE, error in (no error)=w644) -> (queue out=w665:refnum<queue>, error out=w668:errorcluster)  [unwired: 2 in, 1 out]
            n213 = Obtain Queue(name (unnamed)="Script_Info", element data type=w669, error in (no error)=w668) -> (queue out=w671:refnum<queue>, error out=w662:errorcluster)  [unwired: 2 in, 1 out]
            n214 = while {
              tunnel: w671 -> [w683]
              shift-right: [w676] -> w659
              shift-left: w662 -> [w679]
              tunnel: [w682] -> w670
              tunnel: w665 -> [w680]
              tunnel: [w675] -> w663
              stop <- w681 stop-if-true
              n215 = Dequeue Element(queue=w683, error in (no error)=w679) -> (queue out=w682:refnum<queue>, element=w674:T33, error out=w678:errorcluster)  [unwired: 1 in, 1 out]
              "Script Info" <- w674
              n216 = Unbundle By Name(w674) -> ("Done?"=w681:bool)
              n217 = case shown="False" "stop script" {
                selector: "stop script" -> [_ w686]
                tunnel: w680 -> [w685 w690]
                tunnel: w679 -> [w684 w689]
                tunnel: [w684 w688] -> w677
                tunnel: [w685 w687] -> w675
                frame False {
                }
                frame True {
                  n218 = Enqueue Element(queue=w690, element=w686, error in (no error)=w689) -> (queue out=w687:refnum<queue>, error out=w688:errorcluster)  [unwired: 1 in, 1 out]
                }
              }
              n219 = Merge Errors(w677, w678) -> (w676:errorcluster)
            }
            n220 = call "GEA2 Script Test SLB.vi"("GEA2 Reference In"=w657, "Version Query (for log header)"=w661, "Enqueue Sends?"=TRUE, "Standalone"=FALSE, "Script path"="Script Path", "Log File Path (empty for prompt)"="Script Log Path", "Error In"=w662) -> ("Pass/Fail?"=→"Script Pass/Fail?":bool, "Report Text"=→"Script Report Text":string, "Error Out"=→"Script Error Out":errorcluster)  [unwired: 5 in, 1 out]
            n221 = Release Queue(queue=w670, error in (no error)=w659) -> (error out=w664:errorcluster)  [unwired: 1 in, 2 out]
            n222 = Release Queue(queue=w663, error in (no error)=w664) -> (error out=w649:errorcluster)  [unwired: 1 in, 2 out]
            n223 = Enqueue Element(queue=w643, element=T42 {"Data"=variant, "State"=enum."Init"} ("Data"), error in (no error)=w649) -> (error out=w648:errorcluster)  [unwired: 1 in, 2 out]
          }
          event Value Change {
            # "Load Control"
            n224 = event-data() -> ("CtlRef"=w693:refnum<vi>)  [unwired: 1 in, 5 out]
            n225 = property class="Bool"(reference=w693, error in=w694) -> (reference out=w698:refnum<vi>, error out=w699:errorcluster, "Label.Text"=w697:string)
            n226 = Close Reference(reference=w698, error in (no error)=w699) -> (error out=w700:errorcluster)
            n227 = case shown="\"Select Cycle\"" w697 {
              tunnel: w700 -> [w708 w724 w739 w756 w772]
              tunnel: w696 -> [w709 w725 w740 w757 w773]
              tunnel: w695 -> [w707 w723 w738 w755 w771]
              tunnel: [w704 w720 w735 w752 w768] -> w691
              tunnel: [w706 w722 w737 w754 w770] -> w692
              frame "Start Cycle" {
                w701 = T9 {"ERD Number"=62720, "Data Type"=enum."string", "Data"=""}  # ERD Read Data In
                n228 = property on="Cycle Selection" class="DigNum (strict)"(error in=w708) -> (error out=w702:errorcluster, "Value"=w705:u8)  [unwired: 1 in, 1 out]
                n229 = Number To Hexadecimal String(1:i16 2 ("width (-)"), 2:w705) -> (0:w716:string)
                n230 = Concatenate Strings("01" ("string"), w716, "01" ("string")) -> (w714:string)
                n231 = Bundle By Name(cluster=w701, "Data"=w714) -> (w713:T9)
                n232 = Build Array(w713) -> (w711:T9[])
                n233 = call "GEA2 Write ERD.vi"("GEA2 Reference In"=w707, "GEA Inputs"=w709, "Write ERD List"=w711, "Error In"=w702, "Verify ERD Response?"=TRUE) -> ("GEA2 Reference Out"=w704:refnum<k24>, "Error Out"=w706:errorcluster)  [unwired: 8 in, 1 out]
              }
              frame "Stop Cycle", Default {
                w717 = T9 {"ERD Number"=62720, "Data Type"=enum."string", "Data"=""}  # ERD Read Data In
                n234 = property on="Cycle Selection" class="DigNum (strict)"(error in=w724) -> (error out=w718:errorcluster, "Value"=w721:u8)  [unwired: 1 in, 1 out]
                n235 = Number To Hexadecimal String(1:i16 2 ("width (-)"), 2:w721) -> (0:w732:string)
                n236 = Concatenate Strings("01" ("string"), w732, "02" ("string")) -> (w730:string)
                n237 = Bundle By Name(cluster=w717, "Data"=w730) -> (w729:T9)
                n238 = Build Array(w729) -> (w727:T9[])
                n239 = call "GEA2 Write ERD.vi"("GEA2 Reference In"=w723, "GEA Inputs"=w725, "Write ERD List"=w727, "Error In"=w718, "Verify ERD Response?"=TRUE) -> ("GEA2 Reference Out"=w720:refnum<k24>, "Error Out"=w722:errorcluster)  [unwired: 8 in, 1 out]
              }
              frame "Pause Cycle" {
                w745 = T9 {"ERD Number"=62720, "Data Type"=enum."string", "Data"=""}  # ERD Read Data In
                n240 = property on="Cycle Selection" class="DigNum (strict)"(error in=w739) -> (error out=w733:errorcluster, "Value"=w736:u8)  [unwired: 1 in, 1 out]
                n241 = Number To Hexadecimal String(1:i16 2 ("width (-)"), 2:w736) -> (0:w748:string)
                n242 = Concatenate Strings("01" ("string"), w748, "03" ("string")) -> (w746:string)
                n243 = Bundle By Name(cluster=w745, "Data"=w746) -> (w744:T9)
                n244 = Build Array(w744) -> (w742:T9[])
                n245 = call "GEA2 Write ERD.vi"("GEA2 Reference In"=w738, "GEA Inputs"=w740, "Write ERD List"=w742, "Error In"=w733, "Verify ERD Response?"=TRUE) -> ("GEA2 Reference Out"=w735:refnum<k24>, "Error Out"=w737:errorcluster)  [unwired: 8 in, 1 out]
              }
              frame "Resume Cycle" {
                w749 = T9 {"ERD Number"=62720, "Data Type"=enum."string", "Data"=""}  # ERD Read Data In
                n246 = property on="Cycle Selection" class="DigNum (strict)"(error in=w756) -> (error out=w750:errorcluster, "Value"=w753:u8)  [unwired: 1 in, 1 out]
                n247 = Number To Hexadecimal String(1:i16 2 ("width (-)"), 2:w753) -> (0:w764:string)
                n248 = Concatenate Strings("01" ("string"), w764, "04" ("string")) -> (w762:string)
                n249 = Bundle By Name(cluster=w749, "Data"=w762) -> (w761:T9)
                n250 = Build Array(w761) -> (w759:T9[])
                n251 = call "GEA2 Write ERD.vi"("GEA2 Reference In"=w755, "GEA Inputs"=w757, "Write ERD List"=w759, "Error In"=w750, "Verify ERD Response?"=TRUE) -> ("GEA2 Reference Out"=w752:refnum<k24>, "Error Out"=w754:errorcluster)  [unwired: 8 in, 1 out]
              }
              frame "Select Cycle" {
                w765 = T9 {"ERD Number"=62720, "Data Type"=enum."string", "Data"=""}  # ERD Read Data In
                n252 = property on="Cycle Selection" class="DigNum (strict)"(error in=w772) -> (error out=w766:errorcluster, "Value"=w769:u8)  [unwired: 1 in, 1 out]
                n253 = Number To Hexadecimal String(1:i16 2 ("width (-)"), 2:w769) -> (0:w780:string)
                n254 = Concatenate Strings("01" ("string"), w780, "05" ("string")) -> (w778:string)
                n255 = Bundle By Name(cluster=w765, "Data"=w778) -> (w777:T9)
                n256 = Build Array(w777) -> (w775:T9[])
                n257 = call "GEA2 Write ERD.vi"("GEA2 Reference In"=w771, "GEA Inputs"=w773, "Write ERD List"=w775, "Error In"=w766, "Verify ERD Response?"=TRUE) -> ("GEA2 Reference Out"=w768:refnum<k24>, "Error Out"=w770:errorcluster)  [unwired: 8 in, 1 out]
              }
            }
          }
          event "LED Control.ALL LEDs ON", "LED Control.ALL LEDs OFF", "LED Control.Reset LEDs": Value Change {
            # "Load Control Tab"
            n258 = event-data() -> ("CtlRef"=w783:refnum<vi>)  [unwired: 1 in, 5 out]
            n259 = property class="Bool"(reference=w783, error in=w784) -> (reference out=w788:refnum<vi>, error out=w789:errorcluster, "Label.Text"=w787:string)
            n260 = Close Reference(reference=w788, error in (no error)=w789) -> (error out=w790:errorcluster)
            n261 = case shown="\"Reset LEDS\", Default" w787 {
              tunnel: w790 -> [w795 w813 w831]
              tunnel: w786 -> [w796 w814 w829]
              tunnel: w785 -> [w794 w812 w830]
              tunnel: [w793 w811 w828] -> w781
              tunnel: [w792 w810 w827] -> w782
              frame "ALL LEDs ON" {
                w806 = T9 {"ERD Number"=61724, "Data Type"=enum."string", "Data"=""}  # ERD Read Data In
                n262 = Concatenate Strings("0101FFFFFFFFFFFFFFFFFFFF" ("string")) -> (w807:string)
                n263 = Bundle By Name(cluster=w806, "Data"=w807) -> (w805:T9)
                n264 = Build Array(w805) -> (w798:T9[])
                n265 = call "Convert Write ERD List to Message.vi"("GEA Inputs"=w796, "Write ERD List"=w798, "Error In"=w795) -> ("GEA Message"=w800:T21, "Error Out"=w801:errorcluster)  [unwired: 11 in]
                n266 = call "GEA2MessageFormatter.vi"("Prefix(Send/Recv)"="SEND", "GEA2 Data In"=w800, "Error In"=w801) -> ("Output String"=w802:string, "Error Out"=w803:errorcluster)  [unwired: 11 in]
                n267 = call "GExplorer_Queue_GEA2.vi"("Output String"=w802, "error in (no error)"=w803) -> ("error out"=w799:errorcluster)  [unwired: 13 in]
                n268 = call "GEA2 Write ERD.vi"("GEA2 Reference In"=w794, "GEA Inputs"=w796, "Write ERD List"=w798, "Error In"=w799, "Verify ERD Response?"=TRUE) -> ("GEA2 Reference Out"=w793:refnum<k24>, "Error Out"=w792:errorcluster)  [unwired: 8 in, 1 out]
              }
              frame "ALL LEDs OFF" {
                n269 = Concatenate Strings("010100000000000000000000" ("string")) -> (w824:string)
                n270 = Bundle By Name(cluster=T9 {"ERD Number"=61724, "Data Type"=enum."string", "Data"=""} ("ERD Read Data In"), "Data"=w824) -> (w823:T9)
                n271 = Build Array(w823) -> (w816:T9[])
                n272 = call "Convert Write ERD List to Message.vi"("GEA Inputs"=w814, "Write ERD List"=w816, "Error In"=w813) -> ("GEA Message"=w818:T21, "Error Out"=w819:errorcluster)  [unwired: 11 in]
                n273 = call "GEA2MessageFormatter.vi"("Prefix(Send/Recv)"="SEND", "GEA2 Data In"=w818, "Error In"=w819) -> ("Output String"=w820:string, "Error Out"=w821:errorcluster)  [unwired: 11 in]
                n274 = call "GExplorer_Queue_GEA2.vi"("Output String"=w820, "error in (no error)"=w821) -> ("error out"=w817:errorcluster)  [unwired: 13 in]
                n275 = call "GEA2 Write ERD.vi"("GEA2 Reference In"=w812, "GEA Inputs"=w814, "Write ERD List"=w816, "Error In"=w817, "Verify ERD Response?"=TRUE) -> ("GEA2 Reference Out"=w811:refnum<k24>, "Error Out"=w810:errorcluster)  [unwired: 8 in, 1 out]
              }
              frame "Reset LEDS", Default {
                w843 = T9 {"ERD Number"=61724, "Data Type"=enum."string", "Data"=""}  # ERD Read Data In
                n276 = Concatenate Strings("010100000000000000000000" ("string")) -> (w844:string)
                n277 = Bundle By Name(cluster=w843, "Data"=w844) -> (w842:T9)
                n278 = Build Array(w842) -> (w835:T9[])
                n279 = call "Convert Write ERD List to Message.vi"("GEA Inputs"=w829, "Write ERD List"=w835, "Error In"=w831) -> ("GEA Message"=w837:T21, "Error Out"=w838:errorcluster)  [unwired: 11 in]
                n280 = call "GEA2MessageFormatter.vi"("Prefix(Send/Recv)"="SEND", "GEA2 Data In"=w837, "Error In"=w838) -> ("Output String"=w839:string, "Error Out"=w840:errorcluster)  [unwired: 11 in]
                n281 = call "GExplorer_Queue_GEA2.vi"("Output String"=w839, "error in (no error)"=w840) -> ("error out"=w836:errorcluster)  [unwired: 13 in]
                n282 = call "GEA2 Write ERD.vi"("GEA2 Reference In"=w830, "GEA Inputs"=w829, "Write ERD List"=w835, "Error In"=w836, "Verify ERD Response?"=TRUE) -> ("GEA2 Reference Out"=w832:refnum<k24>, "Error Out"=w833:errorcluster)  [unwired: 8 in, 1 out]
                n283 = Concatenate Strings("000000000000000000000000" ("string")) -> (w855:string)
                n284 = Bundle By Name(cluster=T9 {"ERD Number"=61724, "Data Type"=enum."string", "Data"=""} ("ERD Read Data In"), "Data"=w855) -> (w853:T9)
                n285 = Build Array(w853) -> (w846:T9[])
                n286 = call "Convert Write ERD List to Message.vi"("GEA Inputs"=w829, "Write ERD List"=w846, "Error In"=w833) -> ("GEA Message"=w848:T21, "Error Out"=w849:errorcluster)  [unwired: 11 in]
                n287 = call "GEA2MessageFormatter.vi"("Prefix(Send/Recv)"="SEND", "GEA2 Data In"=w848, "Error In"=w849) -> ("Output String"=w850:string, "Error Out"=w851:errorcluster)  [unwired: 11 in]
                n288 = call "GExplorer_Queue_GEA2.vi"("Output String"=w850, "error in (no error)"=w851) -> ("error out"=w847:errorcluster)  [unwired: 13 in]
                n289 = call "GEA2 Write ERD.vi"("GEA2 Reference In"=w832, "GEA Inputs"=w829, "Write ERD List"=w846, "Error In"=w847, "Verify ERD Response?"=TRUE) -> ("GEA2 Reference Out"=w828:refnum<k24>, "Error Out"=w827:errorcluster)  [unwired: 8 in, 1 out]
              }
            }
          }
          event Value Change {
            # "ERD List"
            n290 = event-data() -> ()  [unwired: 1 in, 6 out]
            n291 = Enqueue Element(queue=w858, element=T42 {"Data"=variant, "State"=enum."Build ERD Read List"}, error in (no error)=w860) -> (error out=w859:errorcluster)  [unwired: 1 in, 2 out]
            n292 = call "Write_Header_FGV.vi"("Write Header ? In"=TRUE, "Action"=enum16{"Get", "Set"}."Set", "Error In"=w859) -> ("Error Out"=w862:errorcluster)  [unwired: 11 in, 1 out]
            n293 = call "Select_List.vi"("Load ERD List"="Load ERD List") -> ()  [unwired: 14 in, 1 out]
          }
          event "Clear Fault Seq Buffer": Value Change {
            w878 = T9 {"ERD Number"=57626, "Data Type"=enum."string", "Data"=""}  # ERD Read Data In
            # "Faults Tab"
            n294 = event-data() -> ()  [unwired: 1 in, 6 out]
            n295 = Bundle By Name(cluster=w878, "Data"="01") -> (w877:T9)
            n296 = Build Array(w877) -> (w864:T9[])
            n297 = call "Convert Write ERD List to Message.vi"("GEA Inputs"=w866, "Write ERD List"=w864, "Error In"=w870) -> ("GEA Message"=w873:T21, "Error Out"=w874:errorcluster)  [unwired: 11 in]
            n298 = call "GEA2MessageFormatter.vi"("Prefix(Send/Recv)"="SEND", "GEA2 Data In"=w873, "Error In"=w874) -> ("Output String"=w875:string, "Error Out"=w876:errorcluster)  [unwired: 11 in]
            n299 = call "GExplorer_Queue_GEA2.vi"("Output String"=w875, "error in (no error)"=w876) -> ("error out"=w865:errorcluster)  [unwired: 13 in]
            n300 = call "GEA3 Write ERD (Rev 2 API) Multiple Messages.vi"("GEA2 Reference In"=w867, "GEA Inputs"=w866, "Write ERD List"=w864, "Error In"=w865) -> ("GEA2 Reference Out"=w868:refnum<k24>, "Error Out"=w869:errorcluster)  [unwired: 9 in, 1 out]
          }
          event "Get Faults": Value Change {
            # "Faults Tab"
            n301 = event-data() -> ()  [unwired: 1 in, 6 out]
            n302 = call "Main_Decode_V3.vi"("GEA2 Reference In"=w882, "GEA Inputs"=w886, "Error In"=w885) -> ("Fault Table Status"=w904:T24[], "Major Version"=→"Major Version":u8, "Minor Version"=→"Minor Version":u8, "Fault Table Entries"=w903:T25[][], "GEA2 Reference Out"=w893:refnum<k24>, "Diagnostic Entity Manifest"=w901:T26[], "SnapShot ERD List"=w891:T8[][], "Fault Sequence Status"=w894:T24[], "Fault Sequence Entries"=w902:T23[][], "Error Out"=w892:errorcluster)  [unwired: 5 in, 2 out]
            n303 = Index Array(array=w903) -> (element=w899:T25[])  [unwired: 2 in]
            n304 = Index Array(array=w904) -> (element=w880:T24)  [unwired: 1 in]
            "Fault Table Status" <- w880
            n305 = Index Array(array=w901) -> (element=→"Diagnostic Entity Manifest":T26)  [unwired: 1 in]
            n306 = Index Array(array=w902) -> (element=w896:T23[])  [unwired: 2 in]
            n307 = Index Array(array=w894) -> (element=w889:T24)  [unwired: 1 in]
            "Fault Seq Status" <- w889
            n308 = call "JL_Diag_Filter_Faults.vi"("Filter by Count"="Filter by Count", "Fault Table Entries In"=w899, "Status"=w880) -> ("Fault Table Entries Out"=→"Fault Table Entries":T25[], "Fault Set?"=→"Fault Set?":bool)  [unwired: 11 in]
            n309 = call "JL_Diag_Filter_Seq.vi"("Filter by Count"="Filter by Count", "Fault Table Entries In"=w896, "Status"=w889) -> ("Fault Table Entries Out"=→"Fault Sequence Entries":T23[])  [unwired: 12 in]
            n310 = Unbundle By Name(w880) -> ("Count"=w879:u16)
            n311 = Index Array(array=w891) -> (element=w890:T8[])  [unwired: 2 in]
            n312 = for {
              N: w879 -> [_]
              tunnel: [w913] -> w888 mode=indexing
              tunnel: w886 -> [w911]
              shift-right: [w910] -> w883
              shift-left: w893 -> [w912]
              shift-right: [w908] -> w884
              shift-left: w892 -> [w909]
              tunnel: w890 -> [w907] mode=indexing
              tunnel: "Filter by Count" -> [_]
              n313 = call "JL_Parse_Snapshot.vi"("GEA2 Reference In"=w912, "GEA Inputs"=w911, "SnapShot Location"=w907, "Error In"=w909) -> ("GEA2 Reference Out"=w910:refnum<k24>, "Fault Snapshot"=w913:string[], "Error Out"=w908:errorcluster)  [unwired: 9 in]
            }
            n314 = Transpose 2D Array(2D array=w888) -> (transposed array=→"Centauro Fault Snapshot":string[][])
          }
          event "Clear Fault Table Buffer": Value Change {
            # "Faults Tab"
            n315 = event-data() -> ()  [unwired: 1 in, 6 out]
            n316 = Bundle By Name(cluster=T9 {"ERD Number"=57604, "Data Type"=enum."string", "Data"=""} ("ERD Read Data In"), "Data"="01") -> (w923:T9)
            n317 = Build Array(w923) -> (w921:T9[])
            n318 = call "GEA3 Write ERD (Rev 2 API) Multiple Messages.vi"("GEA2 Reference In"=w920, "# of Tries"=u8 3, "Read Timeout (ms)"=u32 250, "GEA Inputs"=w919, "Write ERD List"=w921, "Error In"=w917) -> ("GEA2 Reference Out"=w918:refnum<k24>, "Error Out"=w916:errorcluster)  [unwired: 7 in, 1 out]
          }
          event "Get Cycle Data": Value Change {
            w925 = T8[] [{"ERD Number"=57661, "Data Type"=enum."string"}, {"ERD Number"=57662, "Data Type"=enum."string"}, {"ERD Number"=57663, "Data Type"=enum."string"}, {"ERD Number"=57664, "Data Type"=enum."string"}, {"ERD Number"=57665, "Data Type"=enum."string"}, {"ERD Number"=57666, "Data Type"=enum."string"}, {"ERD Number"=57667, "Data Type"=enum."string"}, {"ERD Number"=57668, "Data Type"=enum."string"}, {"ERD Number"=57669, "Data Type"=enum."string"}, {"ERD Number"=57670, "Data Type"=enum."string"}, {"ERD Number"=57671, "Data Type"=enum."string"}, {"ERD Number"=57672, "Data Type"=enum."string"}, {"ERD Number"=57673, "Data Type"=enum."string"}, {"ERD Number"=57674, "Data Type"=enum."string"}, {"ERD Number"=57675, "Data Type"=enum."string"}, {"ERD Number"=57676, "Data Type"=enum."string"}, {"ERD Number"=57677, "Data Type"=enum."string"}, {"ERD Number"=57678, "Data Type"=enum."string"}, {"ERD Number"=57679, "Data Type"=enum."string"}, {"ERD Number"=57680, "Data Type"=enum."string"}]
            # "E13D"
            # "Faults Tab"
            # "Erd_DiagnosticsCycleHistorySequenceEntry[0:19]"
            # "Erd_ServiceDiagnosticsCycleHistorySequenceStatus"
            n319 = event-data() -> ()  [unwired: 1 in, 1 out]
            n320 = call "GEA2 Read ERD.vi"("GEA2 Reference In"=w930, "GEA Inputs"=w933, "Read ERD List"=T8[] [{"ERD Number"=57659, "Data Type"=enum."string"}], "Error In"=w929) -> ("GEA2 Reference Out"=w935:refnum<k24>, "ERD Data Out"=w938:T11[], "Error Out"=w934:errorcluster)  [unwired: 8 in, 1 out]
            n321 = Index Array(array=w938) -> (element=w939:T11)  [unwired: 1 in]
            n322 = Unbundle By Name(w939) -> ("Data"=w949:string)
            n323 = call "HexStringToU16.vi"("Input String"=w949, "Starting Offset"=0) -> ("Number Out"=w947:u16)  [unwired: 13 in]
            n324 = call "HexStringToU16.vi"("Input String"=w949, "Starting Offset"=6) -> ("Number Out"=w950:u16)  [unwired: 13 in]
            n325 = call "HexStringToU16.vi"("Input String"=w949, "Starting Offset"=12) -> ("Number Out"=w948:u16)  [unwired: 13 in]
            n326 = Array Size(array=w925) -> (size(s)=w941:i32)
            n327 = Select(t=w950, s="Filter by Status Count", f=w941) -> (s? t:f=w940:i32)
            n328 = Bundle By Name(cluster=T24 {"Cur Index"=0, "Count"=0, "Ov Cnt"=0} ("Fault Table Status"), "Cur Index"=w947, "Count"=w950, "Ov Cnt"=w948) -> (→"output cluster":T24)
            n329 = Array Subset(array=w925, length=w940) -> (w937:T8[])  [unwired: 1 in]
            n330 = for {
              shift-right: [w956] -> w932
              shift-left: w934 -> [w957]
              shift-right: [w954] -> w931
              shift-left: w935 -> [w955]
              tunnel: w937 -> [w953] mode=indexing
              tunnel: w933 -> [w952]
              tunnel: [w951] -> w928 mode=indexing
              n331 = call "JL_Cycle_History_ParseRecord.vi"("Error In"=w957, "Cycle History ERD"=w953, "GEA Inputs"=w952, "GEA2 Reference In"=w955) -> ("Error Out"=w956:errorcluster, "CS2 Dryer"=w951:string[], "GEA2 Reference Out"=w954:refnum<k24>)  [unwired: 3 in, 1 out]
            }
            n332 = Transpose 2D Array(2D array=w928) -> (transposed array=→"JL Cycle History":string[][])
          }
          event "Data ON": Value Change {
            # "Main"
            n333 = event-data() -> ()  [unwired: 1 in, 6 out]
            n334 = case shown="True" "Data ON" {
              tunnel: w961 -> [w964 w968]
              tunnel: [w963 w967] -> w960
              tunnel: w958 -> [w962 w966]
              frame True {
                n335 = Enqueue Element(queue=w962, element=T42 {"Data"=variant, "State"=enum."Init"} ("Data"), error in (no error)=w964) -> (error out=w963:errorcluster)  [unwired: 1 in, 2 out]
              }
              frame False {
                n336 = Enqueue Element(queue=w966, element=T42 {"Data"=variant, "State"=enum."Pause"} ("Data"), error in (no error)=w968) -> (error out=w967:errorcluster)  [unwired: 1 in, 2 out]
              }
            }
          }
          event "Stop": Value Change; User Event; Panel Close {
            # "Main"
            n337 = event-data() -> ()  [unwired: 1 in, 3 out]
            n338 = call "Control_ERD_Loop.vi"("ERD Loop"=w970, "Command (ERD Loop Control)"=ERD_Loop_Control_Command."Shutdown", "Error In"=w979) -> ("Error Out"=w978:errorcluster)  [unwired: 12 in]
            n339 = call "Control_GEA2_Loop.vi"("Command (ERD Loop Control)"=GEA2_Control_Command."Shutdown", "Error In"=w978) -> ("Error Out"=w980:errorcluster)  [unwired: 13 in]
            n340 = call "Control_DAQ_Loop.vi"("Command (DAQ Control)"=DAQ_Control_Command."Shutdown", "Error In"=w980) -> ("Error Out"=w983:errorcluster)  [unwired: 13 in]
            n341 = call "Control_Cont_Send.vi"("Command (ERD Loop Control)"=GEA2_Control_Command."Shutdown", "Error In"=w983) -> ("Error Out"=w972:errorcluster)  [unwired: 13 in]
            n342 = call "Time Delay6"("error in (no error)"=w972, "Delay Time (s)"=1.0) -> ("error out"=w971:errorcluster)  [unwired: 9 in]
          }
          event "Tool Version": Value Change {
            # "Version Tab"
            n343 = event-data() -> ()  [unwired: 1 in, 6 out]
            n344 = property class="App"() -> ("App.Kind"=w986:T51)  [unwired: 2 in, 2 out]
            n345 = case shown="\"Run Time System\"" w986 {
              tunnel: ["invalid" ("File Version Info") w989 w994] -> w987
              frame "invalid app kind", Default {
              }
              frame "Development System", "Student Edition".."Evaluation" {
                n346 = property class="App"() -> ("App.Version"=w989:string)  [unwired: 2 in, 2 out]
              }
              frame "Run Time System" {
                n347 = property class="App"() -> ("App.Dir"=w992:path, "App.Name"=w993:string)  [unwired: 2 in, 2 out]
                n348 = Build Path(base path=w992, name or relative path=w993) -> (appended path=w991:path)
                n349 = call <vilib>:"FileVersionInfo.vi"("Application Path in"=w991) -> ("FileVersionInfo Out"=→"FileVersionInfo":T18, "File Version Info"=w994:string)  [unwired: 7 in, 2 out]
              }
            }
            "LabView/Version Number" <- w987
          }
          event "Get Wifi Data": Value Change {
            n350 = event-data() -> ()  [unwired: 1 in, 6 out]
            n351 = call "Wifi_Data.vi"("GEA2 Reference In"=w1001, "Error In"=w1002) -> ("Wifi Network State"=→"Wifi Network State":string, "GEA2 Reference Out"=w996:refnum<k24>, "Mac Address"=→"Mac Address":string, "Wifi Network Name"=→"Wifi Network Name":string, "Wifi Password"=→"Wifi Password":string, "Error Out"=w995:errorcluster)  [unwired: 8 in]
          }
          event "Residencial": Value Change {
            n352 = event-data() -> ()  [unwired: 1 in, 2 out]
            n353 = call "GEA2 Write ERD.vi"("GEA2 Reference In"=w1016, "GEA Inputs"=w1004, "Write ERD List"=T9[] [{"ERD Number"=65522, "Data Type"=enum."string", "Data"="00"}], "Error In"=w1015) -> ("GEA2 Reference Out"=w1014:refnum<k24>, "Error Out"=w1013:errorcluster)  [unwired: 9 in, 1 out]
            n354 = call "GEA2 Write ERD.vi"("GEA2 Reference In"=w1014, "GEA Inputs"=w1004, "Write ERD List"=T9[] [{"ERD Number"=8397, "Data Type"=enum."string", "Data"="00"}, {"ERD Number"=8398, "Data Type"=enum."boolean", "Data"="00"}, {"ERD Number"=65026, "Data Type"=enum."string", "Data"="00"}, {"ERD Number"=50, "Data Type"=enum."string", "Data"="01"}], "Error In"=w1013) -> ("GEA2 Reference Out"=w1006:refnum<k24>, "Error Out"=w1009:errorcluster)  [unwired: 9 in, 1 out]
            n355 = call "Time Delay7"("error in (no error)"=w1009, "Delay Time (s)"=3.0) -> ("error out"=w1008:errorcluster)  [unwired: 9 in]
            n356 = call "GEA2 Write ERD.vi"("GEA2 Reference In"=w1006, "GEA Inputs"=w1004, "Write ERD List"=T9[] [{"ERD Number"=50, "Data Type"=enum."string", "Data"="01"}], "Error In"=w1008) -> ("GEA2 Reference Out"=w1005:refnum<k24>, "Error Out"=w1007:errorcluster)  [unwired: 9 in, 1 out]
          }
          event "Set Price": Value Change {
            # "00 32 00 32 00 32 00 32 00 00 00 00"
            # "00 19 00 19 00 19 00 19 00 00 00 00"
            # "00 19 00 19 00 19 00 19 00 00 00 00"
            # "DELICATES, LOW, MEDIUM, HIGH"
            # "00 4B 00 64 00 64 00 64 00 00 00 00"
            n357 = event-data() -> ()  [unwired: 1 in, 1 out]
            n358 = call "SetBasePrices.vi"("error in"=w1027, "Cycles"="BasePrices") -> ("error out"=w1026:errorcluster, "PriceData"=w1020:string)  [unwired: 8 in]
            n359 = Bundle By Name(cluster=T9 {"ERD Number"=65529, "Data Type"=enum."string", "Data"=""} ("ERD Write Data In"), "Data"=w1020) -> (w1023:T9)
            n360 = Build Array(w1023) -> (w1022:T9[])
            n361 = call "GEA2 Write ERD.vi"("GEA2 Reference In"=w1032, "GEA Inputs"=w1017, "Write ERD List"=w1022, "Error In"=w1026) -> ("GEA2 Reference Out"=w1031:refnum<k24>, "Error Out"=w1030:errorcluster)  [unwired: 9 in, 1 out]
            n362 = Bundle By Name(cluster=T9 {"ERD Number"=62310, "Data Type"=enum."string", "Data"=""} ("ERD Write Data In"), "Data"=w1020) -> (w1019:T9)
            n363 = Build Array(w1019) -> (w1018:T9[])
            n364 = call "GEA2 Write ERD.vi"("GEA2 Reference In"=w1031, "GEA Inputs"=w1017, "Write ERD List"=w1018, "Error In"=w1030) -> ("GEA2 Reference Out"=w1029:refnum<k24>, "Error Out"=w1028:errorcluster)  [unwired: 9 in, 1 out]
          }
          event "SetIncrementPrices": Value Change {
            n365 = event-data() -> ()  [unwired: 1 in, 1 out]
            n366 = call "SetBasePrices.vi"("error in"=w1040, "Cycles"="IncrementPrices") -> ("error out"=w1046:errorcluster, "PriceData"=w1043:string)  [unwired: 8 in]
            n367 = Bundle By Name(cluster=T9 {"ERD Number"=65530, "Data Type"=enum."string", "Data"=""} ("ERD Write Data In"), "Data"=w1043) -> (w1045:T9)
            n368 = Build Array(w1045) -> (w1036:T9[])
            n369 = call "GEA2 Write ERD.vi"("GEA2 Reference In"=w1038, "GEA Inputs"=w1033, "Write ERD List"=w1036, "Error In"=w1046) -> ("GEA2 Reference Out"=w1048:refnum<k24>, "Error Out"=w1047:errorcluster)  [unwired: 9 in, 1 out]
            n370 = Bundle By Name(cluster=T9 {"ERD Number"=62311, "Data Type"=enum."string", "Data"=""} ("ERD Write Data In"), "Data"=w1043) -> (w1042:T9)
            n371 = Build Array(w1042) -> (w1041:T9[])
            n372 = call "GEA2 Write ERD.vi"("GEA2 Reference In"=w1048, "GEA Inputs"=w1033, "Write ERD List"=w1041, "Error In"=w1047) -> ("GEA2 Reference Out"=w1034:refnum<k24>, "Error Out"=w1035:errorcluster)  [unwired: 9 in, 1 out]
          }
          event "Set Base Time": Value Change {
            # "05 0A 05 05 00 00"
            # "FFFB"
            # "F368"
            n373 = event-data() -> ()  [unwired: 1 in, 1 out]
            n374 = call "SetBaseTime.vi"("error in"=w1058, "Cycles"="Time Base") -> ("error out"=w1056:errorcluster, "TimeData"=w1052:string)  [unwired: 8 in]
            n375 = Bundle By Name(cluster=T9 {"ERD Number"=65531, "Data Type"=enum."string", "Data"=""} ("ERD Write Data In"), "Data"=w1052) -> (w1062:T9)
            n376 = Build Array(w1062) -> (w1053:T9[])
            n377 = call "GEA2 Write ERD.vi"("GEA2 Reference In"=w1055, "GEA Inputs"=w1054, "Write ERD List"=w1053, "Error In"=w1056) -> ("GEA2 Reference Out"=w1064:refnum<k24>, "Error Out"=w1063:errorcluster)  [unwired: 9 in, 1 out]
            n378 = Bundle By Name(cluster=T9 {"ERD Number"=62312, "Data Type"=enum."string", "Data"=""} ("ERD Write Data In"), "Data"=w1052) -> (w1060:T9)
            n379 = Build Array(w1060) -> (w1059:T9[])
            n380 = call "GEA2 Write ERD.vi"("GEA2 Reference In"=w1064, "GEA Inputs"=w1054, "Write ERD List"=w1059, "Error In"=w1063) -> ("GEA2 Reference Out"=w1050:refnum<k24>, "Error Out"=w1049:errorcluster)  [unwired: 9 in, 1 out]
          }
          event "SetTimeIncrement": Value Change {
            # "05 0A 05 05 00 00"
            # "FFFC"
            # "F369"
            n381 = event-data() -> ()  [unwired: 1 in, 1 out]
            n382 = call "SetIncrementTime.vi"("error in"=w1070, "Cycles"="Time Increment") -> ("error out"=w1074:errorcluster, "TimeData"=w1072:string)  [unwired: 8 in]
            n383 = Bundle By Name(cluster=T9 {"ERD Number"=65532, "Data Type"=enum."string", "Data"=""} ("ERD Write Data In"), "Data"=w1072) -> (w1078:T9)
            n384 = Build Array(w1078) -> (w1073:T9[])
            n385 = call "GEA2 Write ERD.vi"("GEA2 Reference In"=w1069, "GEA Inputs"=w1068, "Write ERD List"=w1073, "Error In"=w1074) -> ("GEA2 Reference Out"=w1080:refnum<k24>, "Error Out"=w1079:errorcluster)  [unwired: 9 in, 1 out]
            n386 = Bundle By Name(cluster=T9 {"ERD Number"=62313, "Data Type"=enum."string", "Data"=""} ("ERD Write Data In"), "Data"=w1072) -> (w1076:T9)
            n387 = Build Array(w1076) -> (w1075:T9[])
            n388 = call "GEA2 Write ERD.vi"("GEA2 Reference In"=w1080, "GEA Inputs"=w1068, "Write ERD List"=w1075, "Error In"=w1079) -> ("GEA2 Reference Out"=w1066:refnum<k24>, "Error Out"=w1067:errorcluster)  [unwired: 9 in, 1 out]
          }
          event "Turn off Wifi", "Turn on Wifi": Value Change {
            w1082 = T9 {"ERD Number"=61717, "Data Type"=enum."string", "Data"=""} ("ERD Read Data In")
            n389 = event-data() -> ()  [unwired: 1 in, 6 out]
            n390 = case shown="True" "Turn on Wifi" {
              tunnel: w1087 -> [w1110 w1117]
              tunnel: w1086 -> [w1111 w1116]
              tunnel: w1082 -> [_ w1115]
              tunnel: [w1111 w1113] -> w1084
              tunnel: [w1110 w1114] -> w1085
              tunnel: w1088 -> [w1109 w1112]
              tunnel: [w1109 w1112] -> w1083
              frame False {
              }
              frame True {
                n391 = Concatenate Strings("01" ("string")) -> (w1128:string)
                n392 = Bundle By Name(cluster=w1115, "Data"=w1128) -> (w1127:T9)
                n393 = Build Array(w1127) -> (w1118:T9[])
                n394 = call "Convert Write ERD List to Message.vi"("GEA Inputs"=w1112, "Write ERD List"=w1118, "Error In"=w1116) -> ("GEA Message"=w1122:T21, "Error Out"=w1123:errorcluster)  [unwired: 11 in]
                n395 = call "GEA2MessageFormatter.vi"("Prefix(Send/Recv)"="SEND", "GEA2 Data In"=w1122, "Error In"=w1123) -> ("Output String"=w1124:string, "Error Out"=w1125:errorcluster)  [unwired: 11 in]
                n396 = call "GExplorer_Queue_GEA2.vi"("Output String"=w1124, "error in (no error)"=w1125) -> ("error out"=w1121:errorcluster)  [unwired: 13 in]
                n397 = call "GEA2 Write ERD.vi"("GEA2 Reference In"=w1117, "GEA Inputs"=w1112, "Write ERD List"=w1118, "Error In"=w1121, "Verify ERD Response?"=FALSE) -> ("GEA2 Reference Out"=w1114:refnum<k24>, "Error Out"=w1113:errorcluster)  [unwired: 8 in, 1 out]
              }
            }
            n398 = case shown="True" "Turn off Wifi" {
              tunnel: w1085 -> [w1090 w1097]
              tunnel: w1084 -> [w1091 w1096]
              tunnel: [w1091 w1094] -> _
              tunnel: [w1090 w1095] -> _
              tunnel: w1083 -> [_ w1093]
              tunnel: w1082 -> [_ w1092]
              frame False {
              }
              frame True {
                n399 = Concatenate Strings("02" ("string")) -> (w1108:string)
                n400 = Bundle By Name(cluster=w1092, "Data"=w1108) -> (w1107:T9)
                n401 = Build Array(w1107) -> (w1098:T9[])
                n402 = call "Convert Write ERD List to Message.vi"("GEA Inputs"=w1093, "Write ERD List"=w1098, "Error In"=w1096) -> ("GEA Message"=w1102:T21, "Error Out"=w1103:errorcluster)  [unwired: 11 in]
                n403 = call "GEA2MessageFormatter.vi"("Prefix(Send/Recv)"="SEND", "GEA2 Data In"=w1102, "Error In"=w1103) -> ("Output String"=w1104:string, "Error Out"=w1105:errorcluster)  [unwired: 11 in]
                n404 = call "GExplorer_Queue_GEA2.vi"("Output String"=w1104, "error in (no error)"=w1105) -> ("error out"=w1101:errorcluster)  [unwired: 13 in]
                n405 = call "GEA2 Write ERD.vi"("GEA2 Reference In"=w1097, "GEA Inputs"=w1093, "Write ERD List"=w1098, "Error In"=w1101, "Verify ERD Response?"=FALSE) -> ("GEA2 Reference Out"=w1095:refnum<k24>, "Error Out"=w1094:errorcluster)  [unwired: 8 in, 1 out]
              }
            }
          }
          event "EndOfCycle": Value Change {
            n406 = event-data() -> ()  [unwired: 1 in, 1 out]
            n407 = call "GEA2 Write ERD.vi"("GEA2 Reference In"=w1134, "GEA Inputs"=w1131, "Write ERD List"=T9[] [{"ERD Number"=61467, "Data Type"=enum."string", "Data"="05"}], "Error In"=w1133) -> ("GEA2 Reference Out"=w1130:refnum<k24>, "Error Out"=w1129:errorcluster)  [unwired: 9 in, 1 out]
          }
          event "Set Wifi State(ERD 6003)": Value Change {
            n408 = event-data() -> ()  [unwired: 1 in, 6 out]
            n409 = case shown="\"0 - OFF\", Default" "Wifi State" {
              tunnel: ["00" "01" "02" "03" "04" "05" "06" "FF"] -> w1141
              frame "0 - OFF", Default {
              }
              frame "1 - App Mode" {
              }
              frame "2 - Connecting" {
              }
              frame "3 - Connected" {
              }
              frame "4 - Connected Off" {
              }
              frame "5 - Scanning" {
              }
              frame "6 - Reconnecting" {
              }
              frame "255 - Invalid" {
              }
            }
            n410 = case shown="True" "Set Wifi State(ERD 6003)" {
              tunnel: w1137 -> [w1142 w1147]
              tunnel: w1138 -> [w1143 w1151]
              tunnel: [w1143 w1149] -> w1136
              tunnel: [w1142 w1150] -> w1135
              tunnel: w1141 -> [_ w1148]
              frame False {
              }
              frame True {
                w1144 = T13 {"Source"=228, "Destination"=191} ("GEA Inputs")
                n411 = Concatenate Strings(w1148) -> (w1160:string)
                n412 = Bundle By Name(cluster=T9 {"ERD Number"=24579, "Data Type"=enum."string", "Data"=""} ("ERD Write Data In"), "Data"=w1160) -> (w1159:T9)
                n413 = Build Array(w1159) -> (w1145:T9[])
                n414 = call "Convert Write ERD List to Message.vi"("GEA Inputs"=w1144, "Write ERD List"=w1145, "Error In"=w1151) -> ("GEA Message"=w1155:T21, "Error Out"=w1156:errorcluster)  [unwired: 11 in]
                n415 = call "GEA2MessageFormatter.vi"("Prefix(Send/Recv)"="SEND", "GEA2 Data In"=w1155, "Error In"=w1156) -> ("Output String"=w1157:string, "Error Out"=w1158:errorcluster)  [unwired: 11 in]
                n416 = call "GExplorer_Queue_GEA2.vi"("Output String"=w1157, "error in (no error)"=w1158) -> ("error out"=w1154:errorcluster)  [unwired: 13 in]
                n417 = call "GEA2 Write ERD.vi"("GEA2 Reference In"=w1147, "GEA Inputs"=w1144, "Write ERD List"=w1145, "Error In"=w1154, "Verify ERD Response?"=FALSE) -> ("GEA2 Reference Out"=w1150:refnum<k24>, "Error Out"=w1149:errorcluster)  [unwired: 8 in, 1 out]
              }
            }
          }
          event "Phase.Idle": Value Change {
            n418 = event-data() -> ()  [unwired: 1 in, 1 out]
            n419 = call "GEA2 Write ERD.vi"("GEA2 Reference In"=w1173, "GEA Inputs"=w1169, "Write ERD List"=T9[] [{"ERD Number"=8350, "Data Type"=enum."string", "Data"="FF FF FF FF 00 01 00 03 FF FF FF FF FF FF FF FF FF FF FF FF FF FF FF FF FF FF FF FF F0 00 FF FF"}], "Error In"=w1172) -> ("GEA2 Reference Out"=w1171:refnum<k24>, "Error Out"=w1170:errorcluster)  [unwired: 9 in, 1 out]
          }
          event "Phase.Reserved": Value Change {
            n420 = event-data() -> ()  [unwired: 1 in, 1 out]
            n421 = call "GEA2 Write ERD.vi"("GEA2 Reference In"=w1178, "GEA Inputs"=w1177, "Write ERD List"=T9[] [{"ERD Number"=8350, "Data Type"=enum."string", "Data"="FF FF FF FF 01 01 00 03 FF FF FF FF FF FF FF FF FF FF FF FF FF FF FF FF FF FF FF FF F0 00 FF FF"}], "Error In"=w1179) -> ("GEA2 Reference Out"=w1176:refnum<k24>, "Error Out"=w1175:errorcluster)  [unwired: 9 in, 1 out]
          }
          event "Phase.Authorized": Value Change {
            n422 = event-data() -> ()  [unwired: 1 in, 1 out]
            n423 = call "GEA3 Read ERD (Rev 2 API) Multiple Messages.vi"("GEA2 Reference In"=w1196, "Retry Count"=2, "GEA Inputs"=w1182, "Read ERD List"=cluster{"ERD Number":u16, "Data Type":T10}[] [{"ERD Number"=8351, "Data Type"=enum."string"}], "Error In"=w1195, "Verify ERD Response?"=TRUE) -> ("GEA2 Reference Out"=w1193:refnum<k24>, "ERD Data Out"=w1191:cluster{"ERD Number":u16, "Data":string}[], "Error Out"=w1192:errorcluster)  [unwired: 6 in, 1 out]
            n424 = Array To Cluster(array=w1191) -> (cluster=w1190:T52)
            n425 = Unbundle By Name(w1190) -> ("ERD Data Out[0].Data"=w1189:string)
            n426 = Search and Replace String(input string=w1189, search string="02", replace string="06" ("replace string (\"\")"), offset=4 ("offset (0)")) -> (result string=w1185:string)  [unwired: 4 in, 3 out]
            n427 = Bundle By Name(cluster=T9 {"ERD Number"=8350, "Data Type"=enum."string", "Data"=""} ("ERD Write Data In"), "Data"=w1185) -> (w1184:T9)
            n428 = Build Array(w1184) -> (w1183:T9[])
            n429 = call "GEA2 Write ERD.vi"("GEA2 Reference In"=w1193, "GEA Inputs"=w1182, "Write ERD List"=w1183, "Error In"=w1192) -> ("GEA2 Reference Out"=w1200:refnum<k24>, "Error Out"=w1199:errorcluster)  [unwired: 9 in, 1 out]
          }
          event "See Price": Value Change {
            n430 = event-data() -> ()  [unwired: 1 in, 1 out]
            n431 = call "GEA3 Read ERD (Rev 2 API) Multiple Messages.vi"("GEA2 Reference In"=w1217, "GEA Inputs"=w1211, "Read ERD List"=cluster{"ERD Number":u16, "Data Type":T10}[] [{"ERD Number"=62310, "Data Type"=enum."string"}], "Error In"=w1216) -> ("GEA2 Reference Out"=w1214:refnum<k24>, "ERD Data Out"=w1208:cluster{"ERD Number":u16, "Data":string}[], "Error Out"=w1215:errorcluster)  [unwired: 8 in, 1 out]
            n432 = Array To Cluster(array=w1208) -> (cluster=w1207:T52)
            n433 = Unbundle By Name(w1207) -> ("ERD Data Out[0].Data"=w1206:string)
            n434 = call "Separate_Prices.vi"("Frame"=w1206) -> ("Base Price"=→"Base Price":T14)  [unwired: 10 in]
            n435 = call "GEA3 Read ERD (Rev 2 API) Multiple Messages.vi"("GEA2 Reference In"=w1214, "GEA Inputs"=w1211, "Read ERD List"=cluster{"ERD Number":u16, "Data Type":T10}[] [{"ERD Number"=62311, "Data Type"=enum."string"}], "Error In"=w1215) -> ("GEA2 Reference Out"=w1213:refnum<k24>, "ERD Data Out"=w1202:cluster{"ERD Number":u16, "Data":string}[], "Error Out"=w1212:errorcluster)  [unwired: 8 in, 1 out]
            n436 = Array To Cluster(array=w1202) -> (cluster=w1203:T52)
            n437 = Unbundle By Name(w1203) -> ("ERD Data Out[0].Data"=w1204:string)
            n438 = call "Separate_Prices.vi"("Frame"=w1204) -> ("Base Price"=→"Increment Price":T14)  [unwired: 10 in]
          }
          event "See Times": Value Change {
            n439 = event-data() -> ()  [unwired: 1 in, 1 out]
            n440 = call "GEA3 Read ERD (Rev 2 API) Multiple Messages.vi"("GEA2 Reference In"=w1224, "GEA Inputs"=w1222, "Read ERD List"=cluster{"ERD Number":u16, "Data Type":T10}[] [{"ERD Number"=62312, "Data Type"=enum."string"}], "Error In"=w1223) -> ("GEA2 Reference Out"=w1233:refnum<k24>, "ERD Data Out"=w1230:cluster{"ERD Number":u16, "Data":string}[], "Error Out"=w1234:errorcluster)  [unwired: 8 in, 1 out]
            n441 = Array To Cluster(array=w1230) -> (cluster=w1229:T52)
            n442 = Unbundle By Name(w1229) -> ("ERD Data Out[0].Data"=w1219:string)
            n443 = call "Separate_Times.vi"("Frame"=w1219) -> ("Base Time"=→"Base Time":T15)  [unwired: 9 in, 1 out]
            n444 = call "GEA3 Read ERD (Rev 2 API) Multiple Messages.vi"("GEA2 Reference In"=w1233, "GEA Inputs"=w1222, "Read ERD List"=cluster{"ERD Number":u16, "Data Type":T10}[] [{"ERD Number"=62313, "Data Type"=enum."string"}], "Error In"=w1234) -> ("GEA2 Reference Out"=w1226:refnum<k24>, "ERD Data Out"=w1227:cluster{"ERD Number":u16, "Data":string}[], "Error Out"=w1225:errorcluster)  [unwired: 8 in, 1 out]
            n445 = Array To Cluster(array=w1227) -> (cluster=w1228:T52)
            n446 = Unbundle By Name(w1228) -> ("ERD Data Out[0].Data"=w1221:string)
            n447 = call "Separate_Times.vi"("Frame"=w1221) -> ("Increment Time"=→"Increment Time":T15)  [unwired: 9 in, 1 out]
          }
        }
        n448 = call "Error_Control.vi"("Error In"=w269) -> ("Error Out"=w271:errorcluster)  [unwired: 14 in]
      }
      n449 = call "GEA2 Stop.vi"("GEA2 Reference In"=w64, "Error In"=w65) -> ("Error Out"=w13:errorcluster)  [unwired: 13 in]
      n450 = Close File(refnum=w40, error in=w42) -> (error out=w41:errorcluster)  [unwired: 1 out]
      n451 = Merge Errors(w41, w13, w13, w13, w13, w13) -> (w58:errorcluster)
      n452 = Obtain Queue(name (unnamed)="ERD Loop", element data type=T42 {"Data"=variant, "State"=enum."Read ERDs"} ("Data"), error in (no error)=w58) -> (queue out=w61:refnum<queue>, error out=w60:errorcluster)  [unwired: 2 in, 1 out]
      n453 = Release Queue(queue=w61, error in (no error)=w60) -> (error out=w57:errorcluster)  [unwired: 1 in, 2 out]
      n454 = Merge Errors(w57) -> (w56:errorcluster)
      n455 = call "Error_Control.vi"("Command (Handle Errors)"=Error_Command."Report Errors", "Error In"=w56) -> ("Error Out"=w55:errorcluster)  [unwired: 13 in]
    }
    frame Error {
    }
  }
  n456 = call <vilib>:"Simple Error Handler.vi"("error in (no error)"=w12) -> ("error out"=→"Error Out":errorcluster)  [unwired: 4 in, 4 out]
